vi "2011 Plotter Cole version.vi"() -> ()   [LabVIEW 2011]
uses:
  General-Controler/panel position.ctl
  shared programs/MySQL/Preset Query Enum.ctl
  plotter setup cluster.ctl
  <vilib>/Utility/tcp.llb/UDP Multicast Read-Only Open.vi
  <vilib>/Analysis/1siggen.llb/Ramp Pattern by Samples.vi
  <vilib>/Analysis/NI_AALBase.lvlib
panel:
  in  "STOP button":bool
  out "shot# 3":i32
  out "error out 3":errorcluster
  out "TCP Ports":refnum<k5>[](array[refnum])
  in  "Device name":string
  in  "shot #":i32
  in  "data string":string
  in  "data string 2":string
  in  "shot # 2":i32
  in  "Device name 2":string
  out "subscribe command":string
  out "size(s)":i32
  out "appended array":string[](array[string])
  out "y2":dbl[](array[numeric])
  out "y1":dbl[](array[numeric])
  out "error out 4":errorcluster
  out "x":dbl[](array[numeric])
  out "portrsvvv":string[](array[string])
  out "ipjjj":string[](array[string])
  out "IPs":string[](array[string])
  out "udp ports to listen to":string[](array[string])
  in  "TCP Open timeout ms":i32=1000
  out "TCP scan error out":errorcluster
  out "ScanData to receive":string[][](array[string])
  out "error out":errorcluster
  in  "Cluster":T1
  out "appargs":string[](array[string])
  out "plotter details":string[][](array[string])
  out "plotter#":string
  out "expt":string
  out "expt_plotter.id":string
  out "Mcast Data":string
  out "TDMS file path":path
  in  "Tab Control 2":T2(tab)
  out "parameters to get":string[][](array[string])
  out "devices to get data from":string[](array[string])
  out "Axis Name List":string[](array[string])
  out "All Devices Core Info":string[][](array[string])
  out "UDP Mcast Error":errorcluster
  in  "Tab Control":T3(tab)=enum."Binned Plot"
  out "xy graph":cluster{dbl[], dbl[]}[](graph)
  out "LHS sigma":dbl format="%_4p"
  out "LHS mean":dbl format="%_4p"
  out "RHS mean":dbl format="%_4p"
  out "RHS sigma":dbl format="%_4p"
  out "xy graph bin":cluster{dbl[], dbl[]}[](graph)=[{[5.5, 15.5, 25.5, 35.5, 45.5, 55.5, 0.0], [0.1, 0.1, 0.15, 0.15, 0.2, 0.2, 0.0]}, {[5.5, 5.5, nan, 15.5, 15.5, nan, 25.5, 25.5, nan, 35.5, 35.5, nan, 45.5, 45.5, nan, 55.5, 55.5, nan, 0.0, 0.0, nan], [0.1, 0.1, nan, 0.1, 0.1, nan, 0.15, 0.15, nan, 0.15, 0.15, nan, 0.2, 0.2, nan, 0.2, 0.2, nan, 0.0, 0.0, nan]}, {[5.5, 15.5, 25.5, 35.5, 45.5, 55.5, 0.0], [5.5, 15.5, 25.5, 35.5, 45.5, 55.5, 0.0]}, {[5.5, 5.5, nan, 15.5, 15.5, nan, 25.5, 25.5, nan, 35.5, 35.5, nan, 45.5, 45.5, nan, 55.5, 55.5, nan, 0.0, 0.0, nan], [3.0, 8.0, nan, 13.0, 18.0, nan, 23.0, 28.0, nan, 33.0, 38.0, nan, 43.0, 48.0, nan, 53.0, 58.0, nan, 0.0, 0.0, nan]}]
  in  "replot":bool
  out "Experiment":u16(ring) items=["10TW colliding pulse", "Bella", "FakeCam1only", "FakeCam1to5", "GOG", "Staging", "StagingTRA", "Test stand default", "TREX high power", "TREX low power"]
  out "Current State":string
  out "Mcast Path Data":string
  in  "FilePath":bool
  in  "file path":path
  in  "X Axis":u16(ring)=1 items=["FakeCam1 gain", "FakeCam2 gain", "FakeCam3 gain", "FakeCam4 gain", "FakeCam5 gain"]
  in  "Y Axis":u16(ring) items=["FakeCam1 gain", "FakeCam2 gain", "FakeCam3 gain", "FakeCam4 gain", "FakeCam5 gain"]
  in  "Y Axis 2":u16(ring) items=["FakeCam1 gain", "FakeCam2 gain", "FakeCam3 gain", "FakeCam4 gain", "FakeCam5 gain"]
  out "device data Spreadsheet format":string[][](array[string])
  in  "Left":i16=25
  in  "Top":i16=75
  in  "expt_Plotteridfor vi mode":string="17"
  in  "timeout ms":i32=1000
  out "x axis name":string
  out "ScanStart ExptName":string
  out "Y Axis Default name":string
  out "MC_IP":string
  out "Path used":path
  out "error out 2":errorcluster
  out "ScanStatus":string
  out "data out 1":string
  out "data out 3":string
  out "data out 2":string
  out "shotoverride":bool
  out "shot#":i32
  out "shot# 2":i32
  out "error out 5":errorcluster
  # "Plotter"
  # "17 Fake cam 1 to 5"
  # "15"
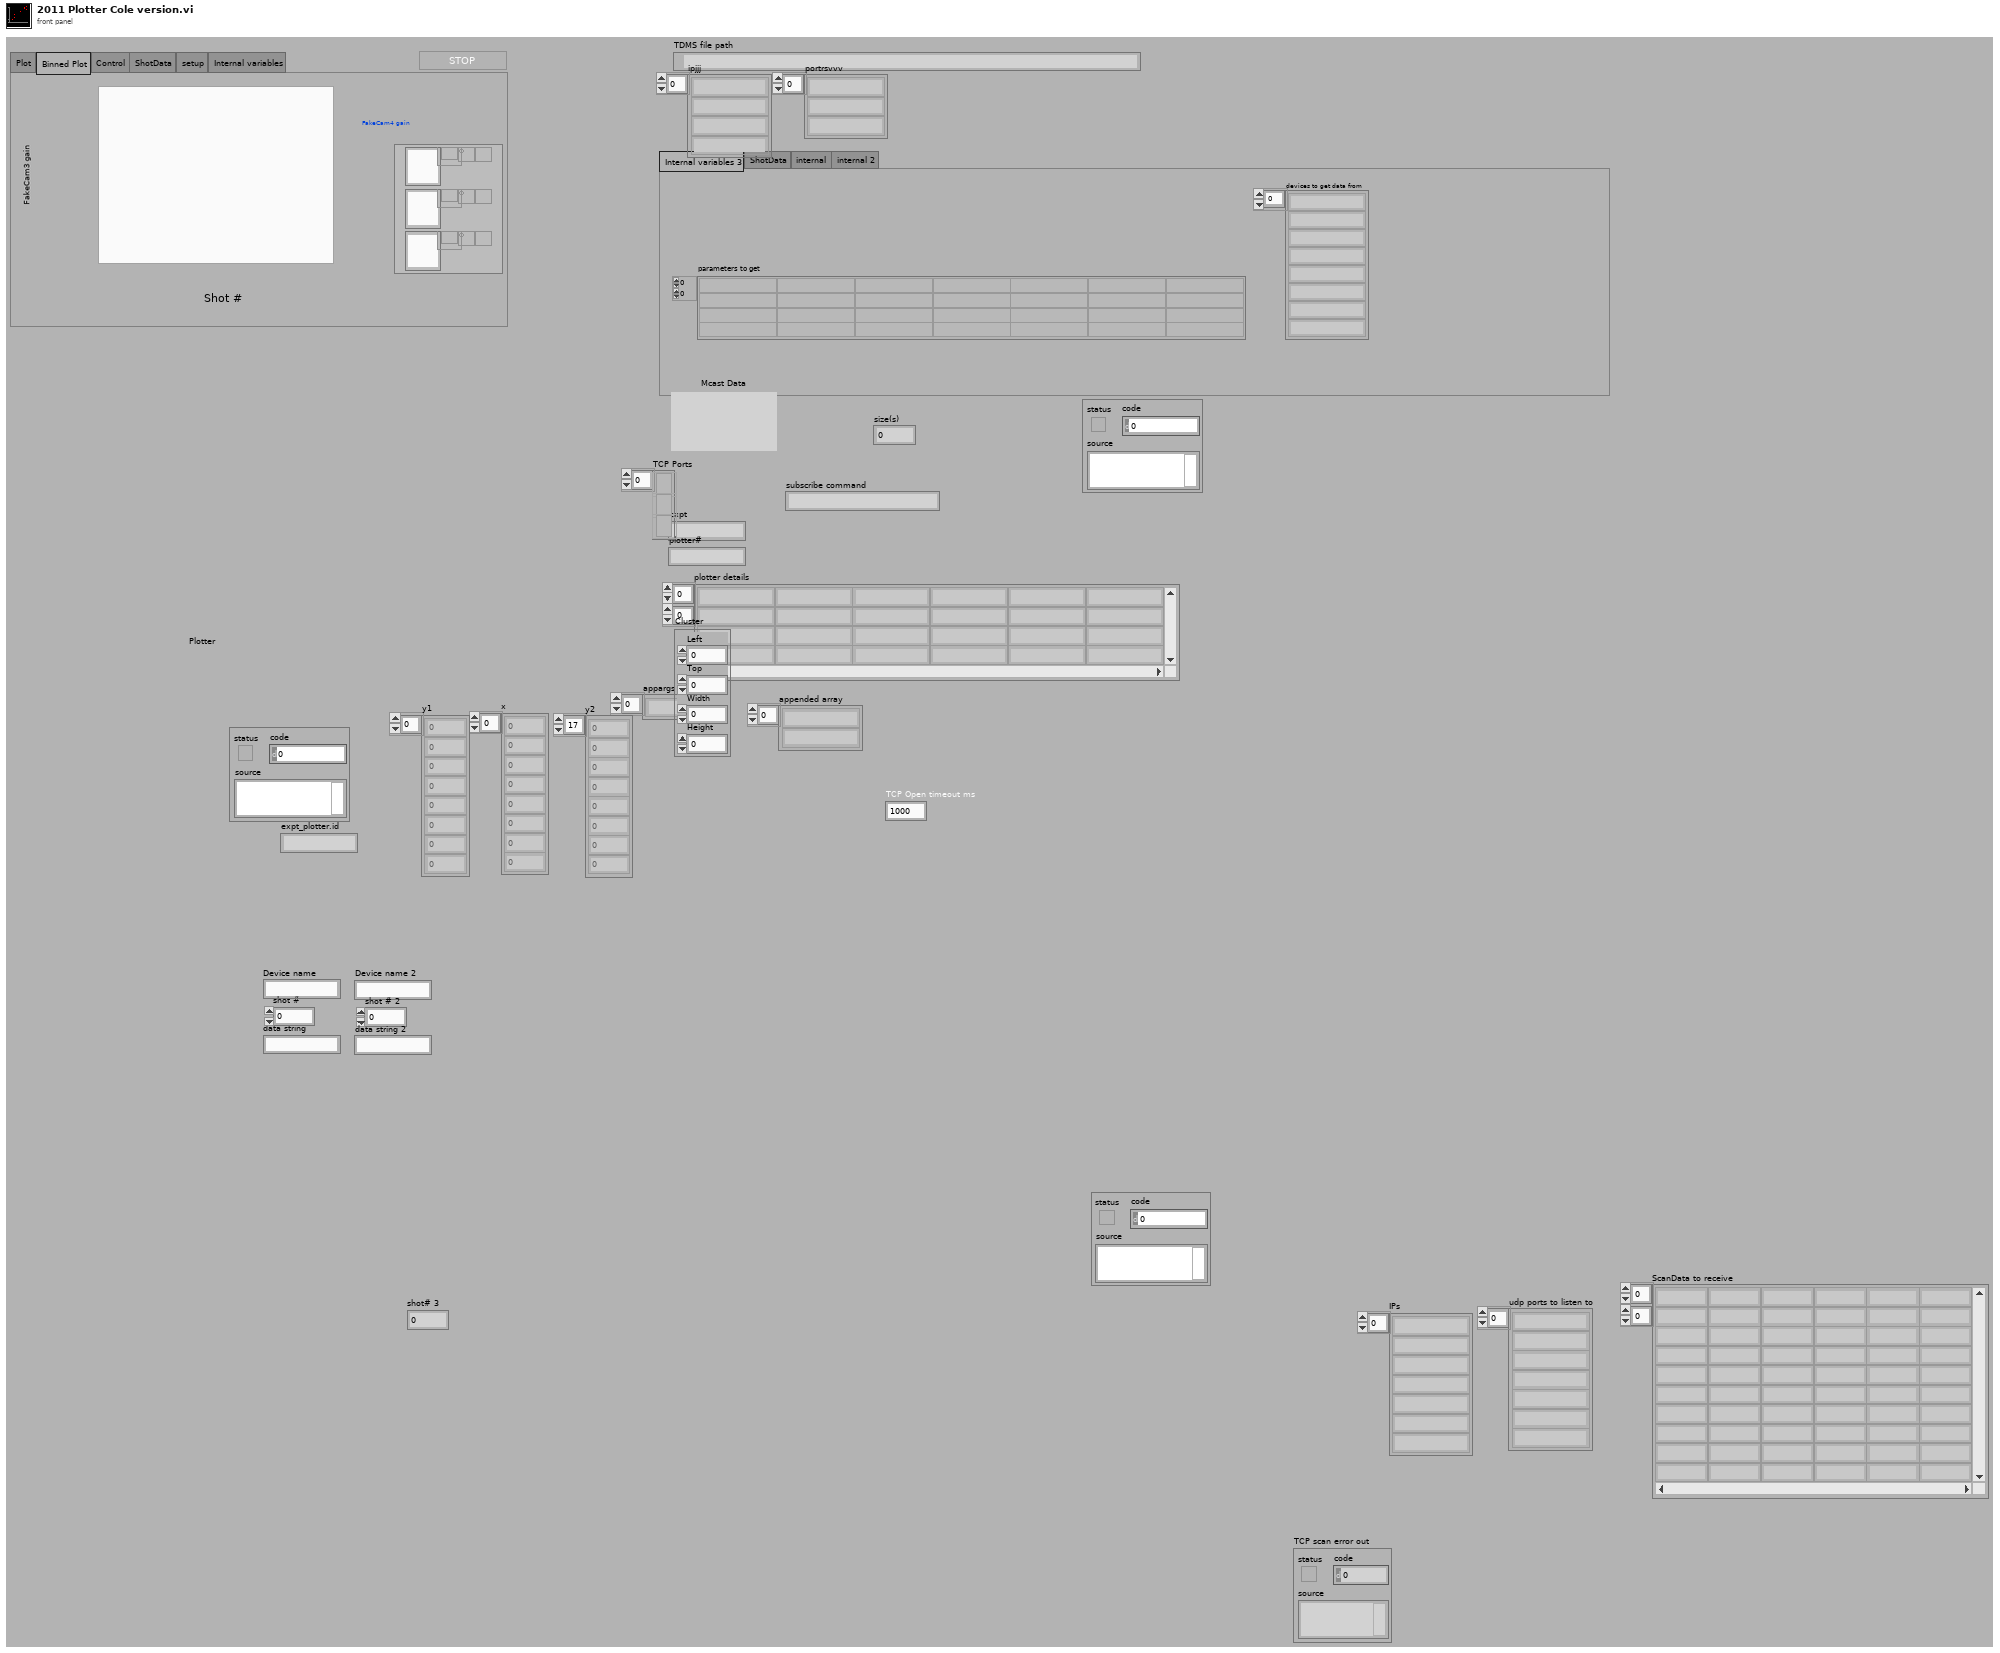
[diagram p1: front panel]
types:
  T1 = typedef "panel position.ctl" = cluster{"Left":i16, "Top":i16, "Width":u32, "Height":u32}
  T2 = enum32{"Internal variables 3", "ShotData", "internal", "internal 2"}
  T3 = enum32{"Plot", "Binned Plot", "Control", "ShotData", "setup", "Internal variables"}
  T4 = typedef "Plotter FGV cluster control.ctl" = cluster{"Multicast Address":string, "Plotter Busy":bool, "Plotter Exit":bool, "Mcast Port":u16}
  T5 = enum32{"invalid app kind", "Development System", "Run Time System", "Student Edition", "Embedded LabVIEW", "Evaluation", "Custom"}
  T6 = enum32{"Invalid", "Standard", "Closed", "Hidden", "Minimized", "Maximized"}
  T7 = typedef "Preset Query Enum.ctl" = enum16{"Get Locations", "Get all IPs and MACs", "Get classes", "Get expt variables to set at scanstart for particular device", "Get expt devices and variables with start values", "Get expt devices and variables (with data to get)", "Get expt devices with data to get", "Get Expt devices and GUIs", "Get all devices basic properties", "Get Virtual Devices Core Info", "Get Expt names", "Get experiment basic properties", "Get MC Ports", "Get device network comm port", "Get devicetype lvclass path", "Get basic device properties", "Get Init Order", "Get all setable variables of a device", "Get all variables of a devicetype", "Get all variables of a device", "Get plotter details", "Get expt for plotter", "Get plotter IDs from expt", "Get all devices", "Get all Virtual Devices", "Get variable and device info for Virtual Device", "GetItemLocatorIP", "Get IPs for GUIs", "Get DeviceType from Device"}
  T8 = typedef "plotter setup cluster.ctl" = cluster{"screenx":i16, "screeny":i16, "variable1":string, "variable2":string}
  T9 = cluster{"Ring Refnum x":refnum<vi>, "Ring Refnum y":refnum<vi>, "Ring Refnum y 2":refnum<vi>, "XY Graph Refnum":refnum<vi>}
  T10 = cluster{"Core":cluster{"Current VI Reference":refnum<vi>, "Close Panel on Exit?":bool}, "All Devices Core Info":string[][], "Expt Config Files":string[], "Experiment name":string, "ScanData to receive":string[][], "Device Names for scan data":string[], "expt config file array":string[][], "Data titles from config array":string[], "TDMS file path":path, "Plotter setup cluster":T8, "plotter#":string, "bin complete":bool}
  T11 = cluster{"TCP Ports":refnum<vi>, "y1":refnum<vi>, "shot#":refnum<vi>, "data out 1":refnum<vi>}
  T12 = cluster{"TCP Ports":refnum<vi>, "y2":refnum<vi>, "shot# 2":refnum<vi>, "data out 2":refnum<vi>}
  T13 = cluster{"TCP Ports":refnum<vi>, "x":refnum<vi>, "shot# 3":refnum<vi>, "data out 3":refnum<vi>}
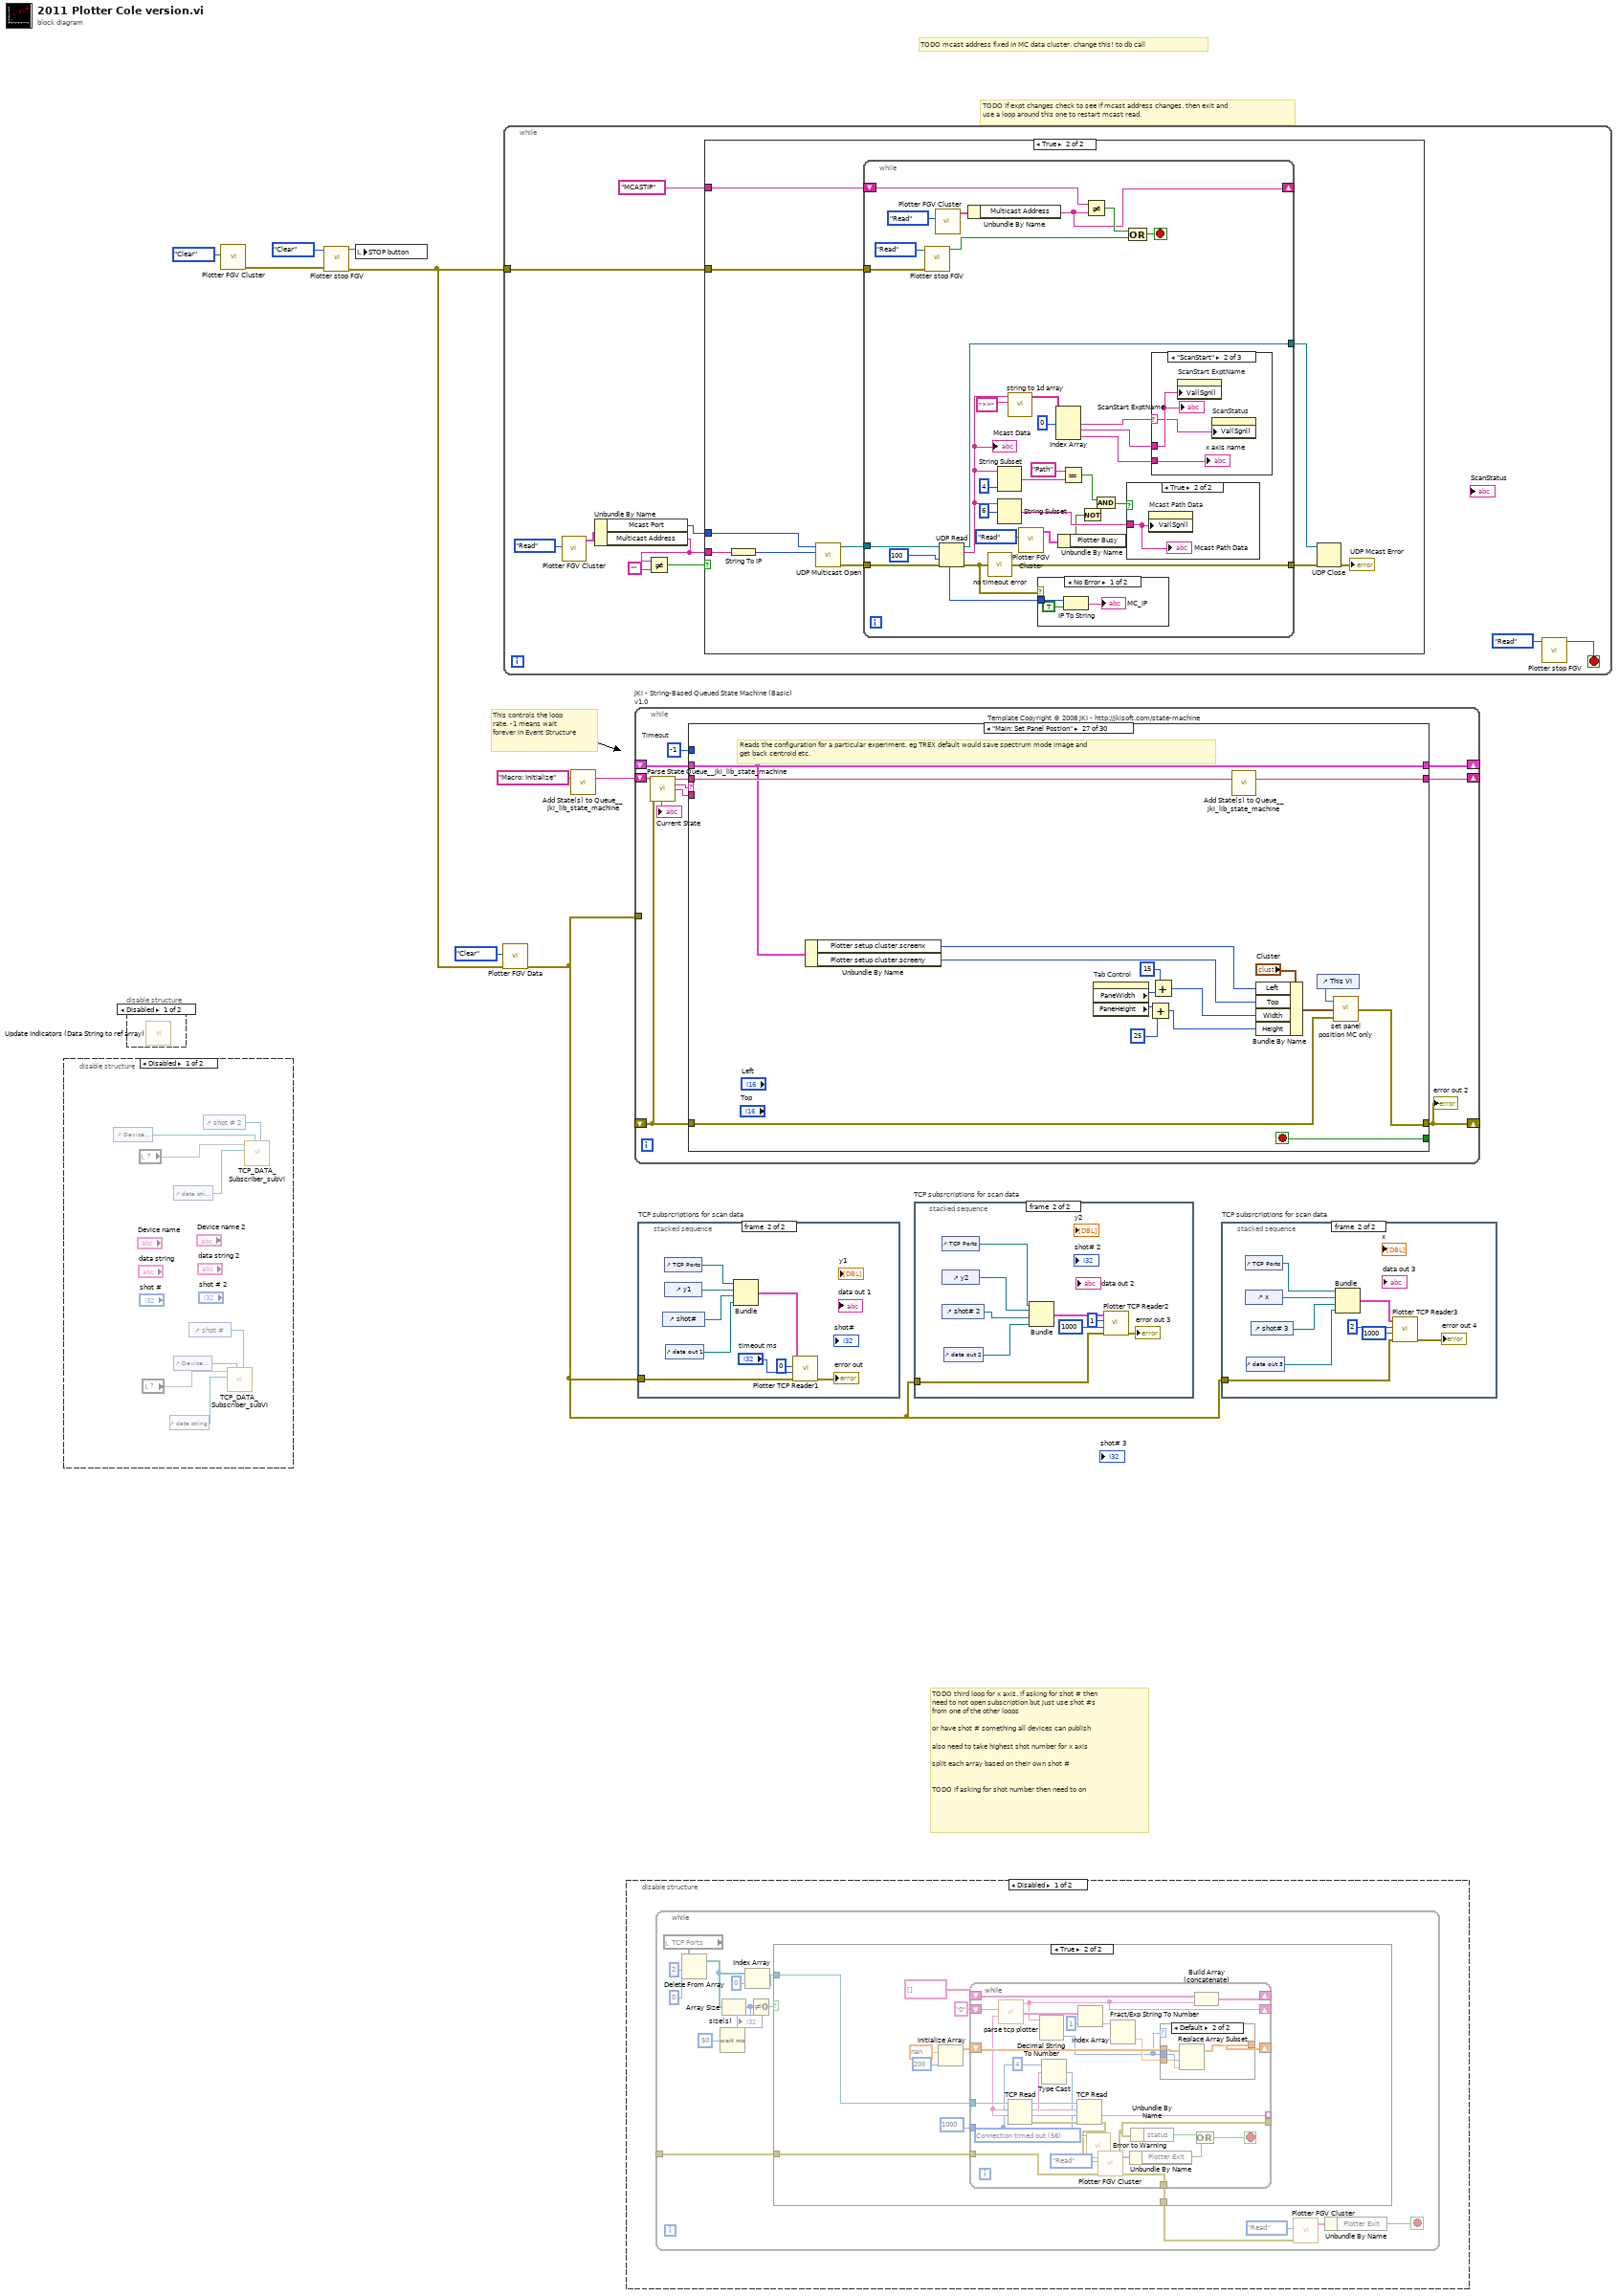
[diagram p0: block diagram]
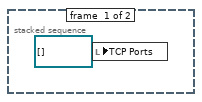
[diagram p5: hidden frame]
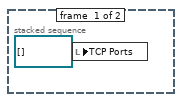
[diagram p6: hidden frame]
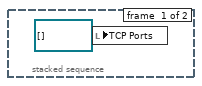
[diagram p8: hidden frame]
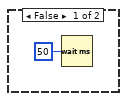
[diagram p10: hidden frame]
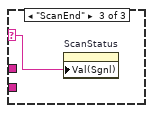
[diagram p14: hidden frame]
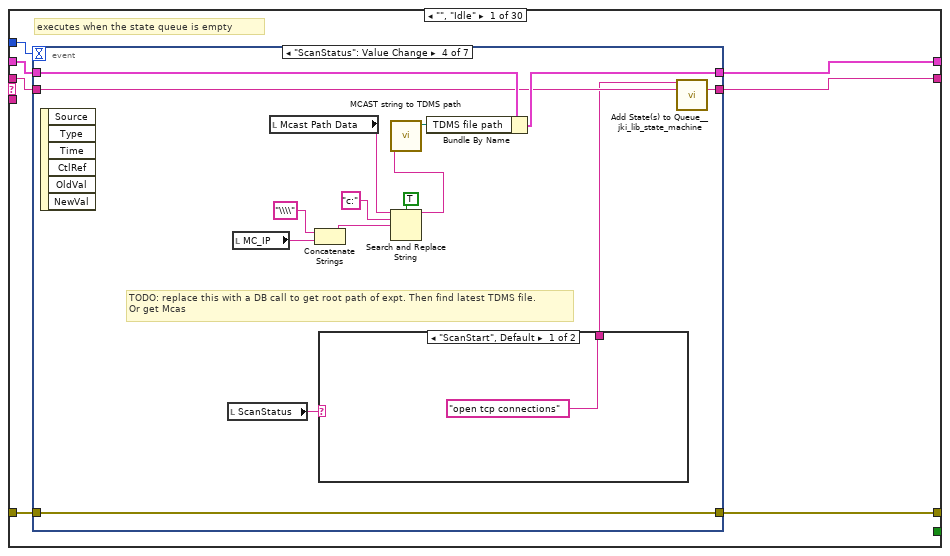
[diagram p15: hidden frame]
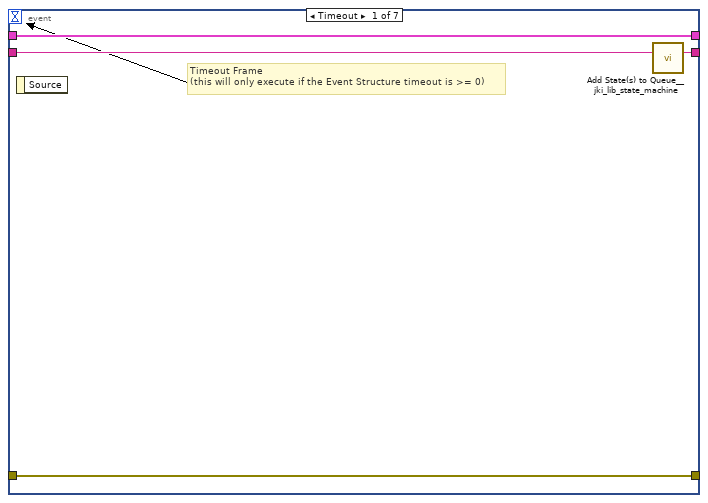
[diagram p16: hidden frame]
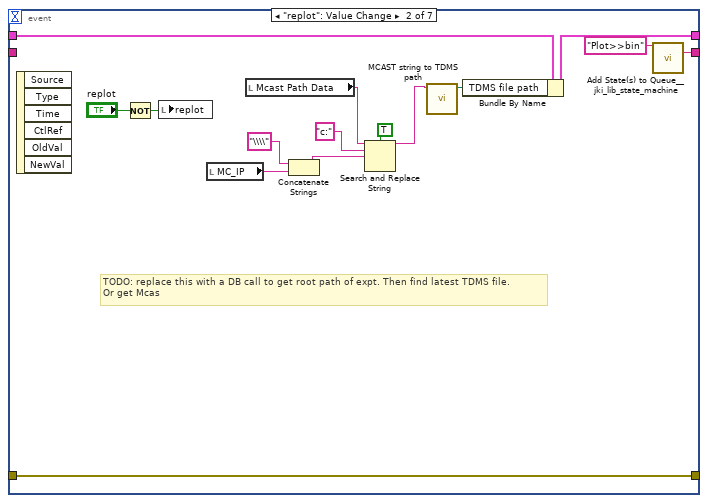
[diagram p17: hidden frame]
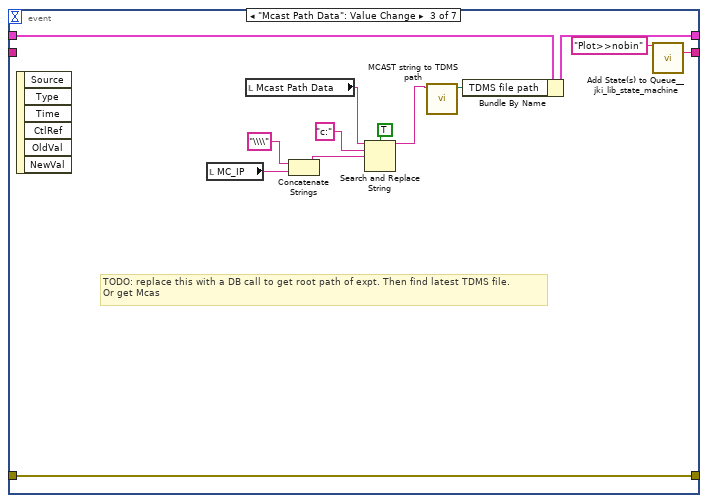
[diagram p18: hidden frame]
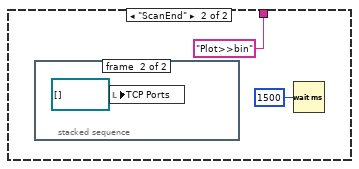
[diagram p19: hidden frame]
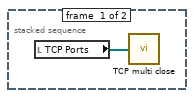
[diagram p20: hidden frame]
diagram:
  # "TODO third loop for x axis. if asking for shot # then \nneed to not open subscription but just use shot #s\nfrom one of the other loops\n\nor have shot # something all devices can publish\n\nalso need to take highest shot number for x axis\n\nsplit each array based on their own shot #\n\n\nTODO if asking for shot number then need to on"
  # "TODO mcast address fixed in MC data cluster. change this! to db call"
  # "TODO if expt changes check to see if mcast address changes. then exit and\nuse a loop around this one to restart mcast read."
  # "This controls the loop rate. -1 means wait forever in Event Structure"
  n1 = disable-structure shown="Disabled" {
    frame Disabled {
      n2 = control-ref of="Device name 2"() -> (w12:refnum<vi>)
      n3 = local read item#-1() -> (w10)
      n4 = local read item#-1() -> (w15)
      n5 = control-ref of="data string"() -> (w14:refnum<vi>)
      n6 = control-ref of="Device name"() -> (w17:refnum<vi>)
      n7 = control-ref of="data string 2"() -> (w11:refnum<vi>)
      n8 = control-ref of="shot #"() -> (w16:refnum<vi>)
      n9 = control-ref of="shot # 2"() -> (w13:refnum<vi>)
      n10 = call "TCP_DATA_Subscriber_subVi.vi"("shot number"=w16, "whatamI"=w17, 10:w14, "connection ID"=w15) -> ()  [unwired: 7 in, 1 out]
      n11 = call "TCP_DATA_Subscriber_subVi.vi"("shot number"=w13, "whatamI"=w12, 10:w11, "connection ID"=w10) -> ()  [unwired: 7 in, 1 out]
    }
    frame Enabled {
    }
  }
  n12 = disable-structure shown="Disabled" {
    frame Disabled {
      n13 = call "Update Indicators (Data String to ref array).vi"() -> ()  [unwired: 5 in, 1 out]
    }
    frame Enabled {
    }
  }
  n14 = call "Plotter FGV Cluster.vi"("Function"=enum16{"Read", "Write", "Clear"}."Clear") -> ("error out"=w5:errorcluster)  [unwired: 9 in, 1 out]
  n15 = call "Plotter stop FGV.vi"("error in"=w5, "Function"=enum16{"Read", "Write", "Clear"}."Clear") -> ("error out"=w2:errorcluster, "Stop out"=w4:bool)  [unwired: 8 in]
  n16 = local write "STOP button"(w4) -> ()
  n17 = call "Plotter FGV Data.vi"("error in"=w2, "Function"=enum16{"Read", "Write", "Clear"}."Clear") -> ("error out"=w1:errorcluster)  [unwired: 8 in, 1 out]
  n18 = while {
    tunnel: w2 -> [w21]
    stop <- w25 stop-if-true
    n19 = call "Plotter FGV Cluster.vi"("Function"=enum16{"Read", "Write", "Clear"}."Read") -> ("Cluster out"=w22:T4)  [unwired: 9 in, 1 out]
    n20 = Unbundle By Name(w22) -> ("Mcast Port"=w18:u16, "Multicast Address"=w20:string)
    n21 = Not Equal?(x=w20, y="") -> (x != y?=w24:bool)
    n22 = case shown="True" w24 {
      tunnel: "MCASTIP" ("Multicast Address") -> [_ w32]
      tunnel: w20 -> [_ w31]
      tunnel: w21 -> [_ w30]
      tunnel: w18 -> [_ w29]
      frame False {
        n23 = Wait (ms)(milliseconds to wait=u32 50) -> ()  [unwired: 1 out]
      }
      frame True {
        n24 = String To IP(1:w31) -> (0:w38:u32)
        n25 = call-poly <vilib>:"UDP Multicast Open.vi"("multicast addr"=w38, "port"=w29) -> ("error out"=w33:errorcluster, "connection ID"=w37:refnum<k16>)  [unwired: 7 in, 1 out]
        n26 = while {
          tunnel: w37 -> [w71]
          tunnel: [w70] -> w36
          tunnel: [w69] -> w35
          tunnel: w33 -> [w65]
          tunnel: w30 -> [w63]
          shift-right: [w39] -> _
          shift-left: w32 -> [w51]
          stop <- w52 stop-if-true
          n27 = call "Plotter stop FGV.vi"("error in"=w63, "Function"=enum16{"Read", "Write", "Clear"}."Read") -> ("Stop out"=w53:bool)  [unwired: 8 in, 1 out]
          n28 = call "Plotter FGV Cluster.vi"("Function"=enum16{"Read", "Write", "Clear"}."Read") -> ("Cluster out"=w50:T4)  [unwired: 9 in, 1 out]
          n29 = UDP Read(connection ID=w71, timeout ms (25000)=100, 8:w65) -> (data out=w54:string, error out=w41:errorcluster, 3:w70:refnum<k16>, 6:w42:u32)  [unwired: 2 out]
          "Mcast Data" <- w54
          n30 = Unbundle By Name(w50) -> ("Multicast Address"=w39:string)
          n31 = call "no timeout error.vi"("error in (no error)"=w41) -> ("error out"=w69:errorcluster)
          n32 = String Subset(string=w54, length (rest)=4 ("length (rest)")) -> (substring=w60:string)  [unwired: 1 in]
          n33 = String Subset(string=w54, offset (0)=6) -> (substring=w58:string)  [unwired: 1 in]
          n34 = call "string to 1d array.vi"("delimiter (Tab)"=">>", "string"=w54) -> ("Array of Strings"=w67:string[])  [unwired: 9 in]
          n35 = call "Plotter FGV Cluster.vi"("Function"=enum16{"Read", "Write", "Clear"}."Read") -> ("Cluster out"=w45:T4)  [unwired: 9 in, 1 out]
          n36 = case shown="No Error" w41 {
            tunnel: w42 -> [w75 _]
            frame No Error {
              n37 = IP To String(1:TRUE ("dot notation? (F)"), 2:w75) -> (0:→"MC_IP":string)
            }
            frame Error {
            }
          }
          n38 = Index Array(array=w67, index #1=0 ("index")) -> (element #1=w48:string, element #2=w55:string, element #3=w56:string)  [unwired: 2 in]
          n39 = Unbundle By Name(w45) -> ("Plotter Busy"=w44:bool)
          n40 = Equal?(x="Path" ("y"), y=w60) -> (x = y?=w57:bool)
          n41 = Not(x=w44) -> (.not. x?=w43:bool)
          n42 = Not Equal?(x=w51, y=w39) -> (x != y?=w40:bool)
          n43 = And(x=w57, y=w43) -> (x .and. y?=w47:bool)
          n44 = case shown="True" w47 {
            tunnel: w58 -> [_ w76]
            frame False {
            }
            frame True {
              n45 = property on="Mcast Path Data" class="Str"("Val(Sgnl)"=w76) -> ()  [unwired: 2 in, 2 out]
              "Mcast Path Data" <- w76
            }
          }
          n46 = Compound Arithmetic op=OR(w40, w53) -> (w52:bool)
          n47 = case shown="\"ScanStart\"" w48 {
            selector: w48 -> [_ w77 w80]
            tunnel: w56 -> [_ w79 _]
            tunnel: w55 -> [_ w78 _]
            frame Default {
            }
            frame "ScanStart" {
              n48 = property on="ScanStart ExptName" class="Str"("Val(Sgnl)"=w78) -> ()  [unwired: 2 in, 2 out]
              n49 = property on="ScanStatus" class="Str"("Val(Sgnl)"=w77) -> ()  [unwired: 2 in, 2 out]
              "x axis name" <- w79
              "ScanStart ExptName" <- w78
            }
            frame "ScanEnd" {
              n50 = property on="ScanStatus" class="Str"("Val(Sgnl)"=w80) -> ()  [unwired: 2 in, 2 out]
            }
          }
        }
        n51 = UDP Close(connection ID=w36, 8:w35) -> (error out=→"UDP Mcast Error":errorcluster)  [unwired: 1 out]
      }
    }
    n52 = call "Plotter stop FGV.vi"("Function"=enum16{"Read", "Write", "Clear"}."Read") -> ("Stop out"=w25:bool)  [unwired: 9 in, 1 out]
  }
  n53 = call <vilib>:"Add State(s) to Queue__jki_lib_state_machine.vi"("State(s) in (\"\")"="Macro: Initialize") -> ("States Out"=w9:string)  [unwired: 14 in]
  n54 = disable-structure shown="Disabled" {
    frame Disabled {
      n55 = while {
        tunnel: _ -> [w87]
        stop <- w88 stop-if-true
        n56 = local read "TCP Ports"() -> (w91:refnum<k5>[])
        n57 = Delete From Array(array=w91, length=2, index=0) -> (array with subset deleted=w83:refnum<k5>[])  [unwired: 1 out]
        n58 = Wait (ms)(milliseconds to wait=u32 50) -> ()  [unwired: 1 out]
        n59 = Array Size(array=w83) -> (size(s)=w94:i32)
        "size(s)" <- w94
        n60 = Index Array(array=w83, index=0) -> (element=w86:refnum<k5>)
        n61 = Not Equal To 0?(x=w94) -> (x != 0?=w93:bool)
        n62 = case shown="True" w93 {
          tunnel: w86 -> [_ w102]
          tunnel: w87 -> [_ w101]
          tunnel: [_ w100] -> w81
          frame False {
          }
          frame True {
            n63 = Initialize Array(nan ("element"), 200 ("dimension size")) -> (w95:dbl[])
            n64 = while {
              tunnel: [w113] -> _
              tunnel: w102 -> [w131]
              tunnel: 1000 ("timeout ms 3") -> [w129]
              tunnel: [w104] -> _ mode=indexing
              shift-right: [w112] -> _
              shift-left: "0" ("shot #") -> [w123]
              tunnel: w101 -> [w119]
              tunnel: [w118] -> w100
              shift-right: [w110] -> _
              shift-left: string[] [] -> [w111]
              shift-right: [w106] -> _
              shift-left: w95 -> [w108]
              stop <- w125 stop-if-true
              w115 = 56 items=["No Error", "Argument Error", "Memory Full", "Out of Zone", "End of File", "File Already Open", "Generic File IO Error", "File Not Found", "File Permission Error", "Disk Full", "Duplicate Path", "Too Many Files Open", "Not Enabled", "Resource File Not Found", "Cannot Add Resource", "Resource Not Found", "Image Not Found", "Image Memory Error", "Pen Does Not Exist", "Config Bad Type", "Config Token Not Found", "Config Parse Error", "Config Memory Error", "Bad External Code Format", "Bad External Code Offset", "External Code Not Present", "Null Window", "Destroy Window Mixup", "Null Menu", "Print Aborted", "Bad Print Record", "Print Driver Error", "Windows Error During Print", "Memory Error During Print", "Print Dialog Error", "Generic Print Error", "Invalid Device Refnum", "Device Not Found", "Device Parameter Error", "Device Unit Error", "Can't Open Device", "Device Call Aborted", "Generic Error", "Cancelled By User", "Object ID Too Low", "Object ID Too High", "Object Not In Heap", "Unknown Heap", "Bad DefProc ID", "DefProc Not In Table", "Message Out Of Range", "Null Method", "Unknown Message", "Manager Call Not Supported", "Bad address", "Connection In progress", "Connection timed out", "Connection is already in progress", "Network attribute not supported", "Network error", "Address in use", "System out of memory", "Connection aborted", "Connection refused", "Connection is not connected", "Connection is already connected", "Connection closed", "Initialize error (interapplication manager)", "Bad occurrence", "Wait on unbound occurrence handler", "Occurrence queue overflow", "Bad path", "Semaphore not signaled", "Unrecognized type (interapplication manager)"] ("1st Error to Convert")
              w128 = 4 ("bytes to read")
              n65 = TCP Read(connection ID=w131, bytes to read=w128, 9:w129) -> (connection ID out=w132:refnum<k5>, data out=w127:string, error out=w130:errorcluster)  [unwired: 2 in]
              n66 = Type Cast(type=w128, x=w127) -> (*(type *) &x=w126:i32)
              n67 = TCP Read(connection ID=w132, bytes to read=w126, error in (no error)=w130, 9:w129) -> (data out=w104:string, error out=w114:errorcluster)  [unwired: 1 in, 1 out]
              n68 = call "parse tcp plotter.vi"("data in"=w104, "shot #"=w123) -> ("variable values"=w117:string[], "shot # out"=w112:string)  [unwired: 8 in]
              n69 = Decimal String To Number(string=w112) -> (number=w105:i32)  [unwired: 2 in, 1 out]
              n70 = Index Array(array=w117, index=1) -> (element=w116:string)
              n71 = call <vilib>:"Error to Warning.vi"("1st Error to Convert"=w115, "error in"=w114) -> ("warning out"=w113:errorcluster)  [unwired: 13 in]
              n72 = call "Plotter FGV Cluster.vi"("error in"=w119, "Function"=enum16{"Read", "Write", "Clear"}."Read") -> ("error out"=w118:errorcluster, "Cluster out"=w121:T4)  [unwired: 8 in]
              n73 = Fract/Exp String To Number(string=w116) -> (number=w107:dbl)  [unwired: 3 in, 1 out]
              n74 = Unbundle By Name(w121) -> ("Plotter Exit"=w120:bool)
              n75 = Unbundle By Name(w113) -> ("status"=w124:bool)
              n76 = case shown="Default" w105 {
                tunnel: w108 -> [w133 w137]
                tunnel: w105 -> [_ w136]
                tunnel: w107 -> [_ w135]
                tunnel: [w133 w134] -> w106
                frame 0 {
                }
                frame Default {
                  n77 = Replace Array Subset(array=w137, new element=w135, index=w136) -> (w134:dbl[])
                }
              }
              n78 = Or(x=w124, y=w120) -> (x .or. y?=w125:bool)
              n79 = Build Array (concatenate)(w111, w112) -> (w110:string[])
            }
          }
        }
        n80 = call "Plotter FGV Cluster.vi"("error in"=w81, "Function"=enum16{"Read", "Write", "Clear"}."Read") -> ("Cluster out"=w90:T4)  [unwired: 8 in, 1 out]
        n81 = Unbundle By Name(w90) -> ("Plotter Exit"=w88:bool)
      }
    }
    frame Enabled {
    }
  }
  n82 = while "JKI - String-Based Queued State Machine (Basic) v1.0" {
    shift-right: [w142] -> _
    shift-left: _ -> [w141]
    shift-right: [w138] -> _
    shift-left: _ -> [w139]
    shift-right: [w144] -> _
    shift-left: w9 -> [w145]
    tunnel: w1 -> [_]
    stop <- w143 stop-if-true
    w140 = -1  # Timeout
    # "Template Copyright © 2008 JKI - http://jkisoft.com/state-machine"
    n83 = call <vilib>:"Parse State Queue__jki_lib_state_machine.vi"("State Queue"=w145, "Error In (no error)"=w139) -> ("Remaining States"=w147:string, "Current State"=w148:string, "Arguments"=w146:string)  [unwired: 11 in]
    "Current State" <- w148
    n84 = case shown="\"Main: Set Panel Postion\"" w148 {
      selector: w148 -> [_ _ _ w247 _ _ _ _ _ _ _ _ _ _ _ _ _ _ _ _ _ _ _ _ _ _ _ _ _ _]
      tunnel: w147 -> [w155 w242 w246 w251 w269 w276 w281 w285 w289 w295 w299 w303 w309 w320 w346 w351 w361 w365 w371 w380 w400 w428 w457 w470 w486 w501 w574 w582 w607 w694]
      tunnel: w146 -> [_ _ _ _ _ _ _ _ _ _ _ _ w304 w314 _ _ _ _ _ _ _ _ _ _ _ _ _ _ w584 _]
      tunnel: w141 -> [w153 w239 w243 w249 w260 w273 w279 w282 _ w290 w296 w301 w307 w316 w343 w347 w359 w362 w368 w377 w398 w414 w455 w463 w483 w499 w568 w579 w605 w691]
      tunnel: [w152 w240 w244 w253 w266 errorcluster {"status"=FALSE, "code"=0, "source"=""} ("error out") w278 w283 w287 w291 w297 w300 w305 w317 w344 w349 w352 w363 w369 w372 w386 w410 w446 w468 w484 w497 w559 w575 w585 w692] -> w138
      tunnel: w139 -> [w151 w240 w244 w252 w266 w270 w278 w283 w287 w292 w297 w300 w306 w318 w344 w349 w352 w363 w369 w373 w387 w411 w436 w468 w484 w498 w560 w576 w586 w692]
      tunnel: [w154 w241 w245 w250 w268 w275 w280 w284 w288 w294 w298 w302 w308 w319 w345 w350 w360 w364 w370 w379 w399 w427 w456 w469 w485 w500 w573 w581 w606 w693] -> w144
      tunnel: [_ _ _ _ _ _ TRUE _ _ _ _ _ _ _ _ _ _ _ _ _ _ _ _ _ _ _ _ _ _ _] -> w143
      tunnel: [w150 w239 w243 w249 w267 w273 w279 w282 w286 w290 w296 w301 w307 w316 w343 w347 w359 w362 w368 w376 w397 w413 w454 w462 w483 w499 w568 w580 w605 w691] -> w142
      tunnel: w140 -> [w149 _ _ _ _ _ _ _ _ _ _ _ _ _ _ _ _ _ _ _ _ _ _ _ _ _ _ _ _ _]
      frame "", "Idle" {
        # "executes when the state queue is empty"
        n85 = event shown="[3] \"ScanStatus\": Value Change" {
          selector: _ -> [_ _ _ _ _ _ _]
          dyn-events: _ -> [_ _ _ _ _ _ _]
          timeout: w149 -> [_ _ _ _ _ _ _]
          tunnel: w155 -> [w159 _ _ w197 w218 w232 w238]
          tunnel: [w158 w174 w187 w202 w217 w231 w237] -> w154
          tunnel: w153 -> [w156 w171 w184 w200 w209 w229 w235]
          tunnel: [w157 w173 w186 w201 w216 w230 w236] -> w152
          tunnel: w151 -> [w157 w173 w186 w201 w216 w230 w236]
          tunnel: [w156 w170 w183 w199 w208 w229 w235] -> w150
          event Timeout {
            # "Timeout Frame\n(this will only execute if the Event Structure timeout is >= 0)"
            n86 = event-data() -> ()  [unwired: 1 in, 1 out]
            n87 = call <vilib>:"Add State(s) to Queue__jki_lib_state_machine.vi"("State(s) in (\"\")"=w159) -> ("States Out"=w158:string)  [unwired: 14 in]
          }
          event "replot": Value Change {
            # "TODO: replace this with a DB call to get root path of expt. Then find latest TDMS file.\nOr get Mcas"
            n88 = event-data() -> ()  [unwired: 1 in, 6 out]
            n89 = Not(x="replot") -> (.not. x?=w168:bool)
            n90 = local write "replot"(w168) -> ()
            n91 = local read "MC_IP"() -> (w164:string)
            n92 = local read "Mcast Path Data"() -> (w166:string)
            n93 = Concatenate Strings("\\\\" ("string"), w164) -> (w161:string)
            n94 = Search and Replace String(case sensitive?=TRUE ("ignore case? (F)"), input string=w166, search string="c:" ("string"), replace string=w161) -> (result string=w160:string)  [unwired: 4 in, 3 out]
            n95 = call "MCAST string to TDMS path.vi"("MCAST path"=w160) -> ("TDMS path"=w167:path)  [unwired: 10 in]
            n96 = Bundle By Name(cluster=w171, "TDMS file path"=w167) -> (w170:T10)
            n97 = call <vilib>:"Add State(s) to Queue__jki_lib_state_machine.vi"("State(s) in Front (\"\")"="Plot>>bin" ("State(s) in Front (\"\")")) -> ("States Out"=w174:string)  [unwired: 14 in]
          }
          event "Mcast Path Data": Value Change {
            # "TODO: replace this with a DB call to get root path of expt. Then find latest TDMS file.\nOr get Mcas"
            n98 = event-data() -> ()  [unwired: 1 in, 6 out]
            n99 = local read "MC_IP"() -> (w179:string)
            n100 = local read "Mcast Path Data"() -> (w181:string)
            n101 = Concatenate Strings("\\\\" ("string"), w179) -> (w176:string)
            n102 = Search and Replace String(case sensitive?=TRUE ("ignore case? (F)"), input string=w181, search string="c:" ("string"), replace string=w176) -> (result string=w175:string)  [unwired: 4 in, 3 out]
            n103 = call "MCAST string to TDMS path.vi"("MCAST path"=w175) -> ("TDMS path"=w182:path)  [unwired: 10 in]
            n104 = Bundle By Name(cluster=w184, "TDMS file path"=w182) -> (w183:T10)
            n105 = call <vilib>:"Add State(s) to Queue__jki_lib_state_machine.vi"("State(s) in Front (\"\")"="Plot>>nobin" ("State(s) in Front (\"\")")) -> ("States Out"=w187:string)  [unwired: 14 in]
          }
          event "ScanStatus": Value Change {
            # "TODO: replace this with a DB call to get root path of expt. Then find latest TDMS file.\nOr get Mcas"
            n106 = event-data() -> ()  [unwired: 1 in, 6 out]
            n107 = local read "ScanStatus"() -> (w189:string)
            n108 = local read "MC_IP"() -> (w195:string)
            n109 = local read "Mcast Path Data"() -> (w191:string)
            n110 = Concatenate Strings("\\\\" ("string"), w195) -> (w192:string)
            n111 = case shown="\"ScanStart\", Default" w189 {
              tunnel: ["open tcp connections" ("State(s) in Front (\"\")") "Plot>>bin" ("State(s) in Front (\"\")")] -> w188
              frame "ScanStart", Default {
              }
              frame "ScanEnd" {
                n112 = stacked-sequence {
                  frame #0 {
                    n113 = local read "TCP Ports"() -> (w206:refnum<k5>[])
                    n114 = call "TCP multi close.vi"("TCP Ports"=w206) -> ()
                  }
                  frame #1 {
                    n115 = local write "TCP Ports"(refnum<k5>[] [] ("TCP Ports")) -> ()
                  }
                }
                n116 = Wait (ms)(milliseconds to wait=u32 1500) -> ()  [unwired: 1 out]
              }
            }
            n117 = Search and Replace String(case sensitive?=TRUE ("ignore case? (F)"), input string=w191, search string="c:" ("string"), replace string=w192) -> (result string=w190:string)  [unwired: 4 in, 3 out]
            n118 = call "MCAST string to TDMS path.vi"("MCAST path"=w190) -> ("TDMS path"=w198:path)  [unwired: 10 in]
            n119 = Bundle By Name(cluster=w200, "TDMS file path"=w198) -> (w199:T10)
            n120 = call <vilib>:"Add State(s) to Queue__jki_lib_state_machine.vi"("State(s) in Front (\"\")"=w188, "State(s) in (\"\")"=w197) -> ("States Out"=w202:string)  [unwired: 13 in]
          }
          event "ScanStart ExptName": Value Change {
            w211 = dbl[] [] ("y1")
            n121 = event-data() -> ()  [unwired: 1 in, 6 out]
            n122 = Bundle By Name(cluster=w209, "bin complete"=FALSE) -> (w208:T10)
            n123 = local read "ScanStart ExptName"() -> (w213:string)
            n124 = property on="Experiment" class="Ring (strict)"() -> ("Strings []"=w214:string[])  [unwired: 2 in, 2 out]
            n125 = Search 1D Array(1D array=w214, element=w213) -> (index of element=w212:i32)  [unwired: 1 in]
            n126 = local write "y2"(w211) -> ()
            n127 = local write "y1"(w211) -> ()
            n128 = local write "x"(w211) -> ()
            n129 = local write "Experiment"(w212) -> ()
            n130 = call <vilib>:"Add State(s) to Queue__jki_lib_state_machine.vi"("State(s) in Front (\"\")"="Main: Macro", "State(s) in (\"\")"=w218) -> ("States Out"=w217:string)  [unwired: 13 in]
          }
          event "STOP button": Value Change {
            # "Exit Button Value Change (pressed) Event\n(this executes Macro: Exit to terminate the VI)"
            n131 = event-data() -> ()  [unwired: 1 in, 1 out]
            n132 = call "Plotter stop FGV.vi"("Stop in"="STOP button", "Function"=enum16{"Read", "Write", "Clear"}."Write") -> ("Stop out"=w226:bool)  [unwired: 8 in, 1 out]
            n133 = Not(x=w226) -> (.not. x?=w225:bool)
            n134 = call "Plotter FGV Cluster.vi"("Function"=enum16{"Read", "Write", "Clear"}."Read") -> ("Cluster out"=w221:T4)  [unwired: 9 in, 1 out]
            n135 = Bundle By Name(cluster=w221, "Plotter Exit"=TRUE) -> (w219:T4)
            n136 = local write "STOP button"(w225) -> ()
            n137 = call "Plotter FGV Cluster.vi"("Function"=enum16{"Read", "Write", "Clear"}."Write", "Cluster in"=w219) -> ()  [unwired: 8 in, 2 out]
            n138 = call <vilib>:"Add State(s) to Queue__jki_lib_state_machine.vi"("State(s) in Front (\"\")"="Macro: Exit", "State(s) in (\"\")"=w232) -> ("States Out"=w231:string)  [unwired: 13 in]
          }
          event Panel Close? {
            # "Discard the event because we'll close the front panel ourselves in Macro: Exit"
            # "Close Panel button (pressed) Event\n(this executes Macro: Exit to terminate the VI)"
            n139 = event-data() -> ()  [unwired: 1 in, 1 out]
            n140 = event-data("Discard?"=TRUE) -> ()  [unwired: 1 in, 1 out]
            n141 = call <vilib>:"Add State(s) to Queue__jki_lib_state_machine.vi"("State(s) in Front (\"\")"="Macro: Exit", "State(s) in (\"\")"=w238) -> ("States Out"=w237:string)  [unwired: 13 in]
          }
        }
      }
      frame "Readme" {
        # "For instructions on how to use the JKI State Machine, examples and video tutorials, visit:\nhttp://jkisoft.com/state-machine/\n\nJKI State Machine™\nhttp://jkisoft.com/state-machine/\nCopyright (C) 2005-2008, JKI <info@jkisoft.com>\nALL RIGHTS RESERVED"
        # "copy this to create labels for wires"
        # "System_Label"
        # "State Syntax:\nStateCategory: State >> Argument\nLine Terminator: Line feed\nExample:\nUI: Help >> About\n\nWhere \"UI\" is the state category\nWhere \"Help\" is the state\nWhere \"About\" is the argument\nOther Examples:\nApp Data: Initialize\nUI: Initialize\nHelp >> About\n\nCommenting:\nTo add a comment use \"//\" or \"#\" and all text to the right will be ignored\nCommenting Example:\nUI: Initialize // This initializes the UI\n# This whole line is a comment\n// Another comment line"
        # "Readme"
        n142 = call <vilib>:"Add State(s) to Queue__jki_lib_state_machine.vi"("State(s) in (\"\")"=w242) -> ("States Out"=w241:string)  [unwired: 14 in]
      }
      frame "---------- Core ----------" {
        # "Do not put any code in this frame.\n(it is a separator no-op)"
        n143 = call <vilib>:"Add State(s) to Queue__jki_lib_state_machine.vi"("State(s) in (\"\")"=w246) -> ("States Out"=w245:string)  [unwired: 14 in]
      }
      frame Default {
        w256 = 42 items=["No error", "Argument error", "Memory is full", "Out of zone", "End of file", "File already open", "Generic file I/O error", "File not found", "File permission error", "Disk is full", "Duplicate path", "Too many files open", "System feature not enabled", "Resource file not found", "Cannot add resource", "Resource not found", "Image not found", "Image memory error", "Pen does not exist", "Config type invalid", "Config token not found", "Config parse error", "Config memory error", "Bad external code format", "Bad external code offset", "External code not present", "Null window", "Destroy window error", "Null menu", "Print aborted", "Bad print record", "Print driver error", "Windows error during printing", "Memory error during printing", "Print dialog error", "Generic print error", "Invalid device refnum", "Device not found", "Device parameter error", "Device unit error", "Cannot open device", "Device call aborted", "Generic error", "Cancelled by user", "Object ID too low", "Object ID too high", "Object not in heap", "Unknown heap", "Unknown object (invalid DefProc)", "Unknown object (DefProc not in table)", "Message out of range", "Invalid (null) method", "Unknown message", "Manager call not supported", "Bad address", "Network operation in progress", "Network operation timed out", "Connection is busy", "Network attribute not supported", "Network error", "Address in use", "System out of memory", "Connection aborted", "Connection refused", "Not connected", "Already connected", "Connection closed", "Initialization error (interapplication manager)", "Bad occurrence", "Wait on unbound occurrence handler", "Occurrence queue overflow", "Datalog type conflict", "Unused", "Unrecognized type (interapplication manager)", "Memory corrupt", "Failed to make temporary DLL", "Old CIN version", "Drag socket not found", "Failed to load drop-object", "Failed to register OLE object", "Failed to release OLE object", "Format specifier type mismatch", "Unknown format specifier", "Too few format specifiers", "Too many format specifiers", "Scan failed", "Newer CIN version", "Error converting to variant", "Runtime menu error", "Password tampered", "Variant attribute not found", "Incompatible variant data type", "Event data is not available", "Event Store is not present", "Occurrence is not found", "Event Queue is not created", "Event info is not available", "Refnum passed is NULL", "Error retrieving Class GUID", "Error retrieving CoClass GUID", "Error retrieving TypeLib GUID.", "Bad built application magic bytes.", "Specific driver is different from the specific driver associated with the Logical Name.", "There is no session opened to the class driver.", "Max Error", "MAX - Error with config objects", "MAX - Error loading configuration", "MAX - Group not supported"]
        # "Current State"
        # "Do not delete, rename, or modify this frame.\n(this is used to capture unhandled states and typos)"
        # "Handle mistyped state name (developer tool)"
        n144 = Format Into String(format string="Software Exception: Unhandled State \"%s\"." ("message"), error in=w252, w247) -> (resulting string=w255:string, error out=w254:errorcluster)  [unwired: 1 in]
        n145 = call <vilib>:"Error Cluster From Error Code.vi"("show call chain? (False)"=TRUE, "error in (no error)"=w254, "error message (\"\")"=w255, "error code (0)"=w256) -> ("error out"=w253:errorcluster)  [unwired: 5 in]
        n146 = call <vilib>:"Add State(s) to Queue__jki_lib_state_machine.vi"("State(s) in (\"\")"=w251) -> ("States Out"=w250:string)  [unwired: 14 in]
      }
      frame "Initialize Core Data" {
        # "Do not delete, rename, or modify this frame.\n(this is used to determine panel behavior on exit)"
        # "originally closed?"
        # "exe?"
        # "If panel starts closed or is an EXE, then close it when we exit"
        n147 = property class="VI"() -> ("Front Panel.Open"=w265:bool)  [unwired: 2 in, 2 out]
        n148 = property class="App"() -> ("App.Kind"=w264:T5)  [unwired: 2 in, 2 out]
        n149 = control-ref of="Current VI Reference"() -> (w258:refnum<vi>)
        n150 = Not(x=w265) -> (.not. x?=w262:bool)
        n151 = Equal?(x=w264, y=T5."Run Time System" ("Application:Kind")) -> (x = y?=w261:bool)
        n152 = Or(x=w262, y=w261) -> (x .or. y?=w259:bool)
        n153 = Bundle By Name(cluster=w260, "Core.Current VI Reference"=w258, "Core.Close Panel on Exit?"=w259) -> (w267:T10)
        n154 = call <vilib>:"Add State(s) to Queue__jki_lib_state_machine.vi"("State(s) in (\"\")"=w269) -> ("States Out"=w268:string)  [unwired: 14 in]
      }
      frame "Error Handler" {
        # "Unhandled Error -- Display it"
        # "Handle any errors here.\nYou can also output any states to clean-up after errors occur"
        # "Clear error"
        n155 = Wait (ms)(milliseconds to wait=u32 1500) -> ()  [unwired: 1 out]
        n156 = call <vilib>:"Add State(s) to Queue__jki_lib_state_machine.vi"("State(s) in Front (\"\")"="/* Post Error States", "State(s) in (\"\")"=w276) -> ("States Out"=w275:string)  [unwired: 13 in]
        "error out 5" <- w270
      }
      frame "Exit" {
        # "Do not put any code in this frame.\n(No errors that occur here will be handled.)"
        n157 = call <vilib>:"Add State(s) to Queue__jki_lib_state_machine.vi"("State(s) in (\"\")"=w281) -> ("States Out"=w280:string)  [unwired: 14 in]
      }
      frame "---------- Data ----------" {
        # "Do not put any code in this frame.\n(It is a separator no-op. You can make a copy of this frame to create a new Data frame)"
        n158 = call <vilib>:"Add State(s) to Queue__jki_lib_state_machine.vi"("State(s) in (\"\")"=w285) -> ("States Out"=w284:string)  [unwired: 14 in]
      }
      frame "Data: Initialize" {
        # "Initialize the shift-register data, here.\n(data names are defined by what you wire into the bundle function)"
        n159 = call "Data Cluster Plotter.vi"() -> ("output cluster"=w286:T10)
        n160 = call <vilib>:"Add State(s) to Queue__jki_lib_state_machine.vi"("State(s) in (\"\")"=w289) -> ("States Out"=w288:string)  [unwired: 14 in]
      }
      frame "Data: Cleanup" {
        # "Cleanup any data and references, here.\n(this is called automatically, by the Macro: Exit)"
        n161 = Unbundle By Name(w290) -> ("Core.Current VI Reference"=w293:refnum<vi>)
        n162 = Close Reference(reference=w293, error in (no error)=w292) -> (error out=w291:errorcluster)
        n163 = call <vilib>:"Add State(s) to Queue__jki_lib_state_machine.vi"("State(s) in (\"\")"=w295) -> ("States Out"=w294:string)  [unwired: 14 in]
      }
      frame "---------- UI ----------" {
        # "Do not put any code in this frame.\n(It is a separator no-op. You can make a copy of this frame to create a new UI frame)"
        n164 = call <vilib>:"Add State(s) to Queue__jki_lib_state_machine.vi"("State(s) in (\"\")"=w299) -> ("States Out"=w298:string)  [unwired: 14 in]
      }
      frame "UI: Initialize" {
        # "Initialize the User Interface, here.\n(this is called automatically, by the Macro: Init)"
        n165 = call <vilib>:"Add State(s) to Queue__jki_lib_state_machine.vi"("State(s) in (\"\")"=w303) -> ("States Out"=w302:string)  [unwired: 14 in]
      }
      frame "UI: Cursor Set" {
        # "Argument"
        # "Set and Unset Cursor Busy.\n(Usage: \"UI: Cursor Set >> Busy|Idle\")"
        n166 = case shown="\"Idle\", Default" w304 {
          tunnel: w306 -> [w311 w313]
          tunnel: [w310 w312] -> w305
          frame "Idle", Default {
            n167 = call <vilib>:"Unset Busy.vi"("error in (no error)"=w311) -> ("error out"=w310:errorcluster)  [unwired: 10 in]
          }
          frame "Busy" {
            n168 = call <vilib>:"Set Busy.vi"("error in (no error)"=w313) -> ("error out"=w312:errorcluster)  [unwired: 9 in, 1 out]
          }
        }
        n169 = call <vilib>:"Add State(s) to Queue__jki_lib_state_machine.vi"("State(s) in (\"\")"=w309) -> ("States Out"=w308:string)  [unwired: 14 in]
      }
      frame "UI: Front Panel State" {
        # "Argument"
        # "Set Front Panel Open or Closed\n(Usage: \"UI: Front Panel State >> Open|Close\")"
        n170 = Unbundle By Name(w316) -> ("Core.Current VI Reference"=w315:refnum<vi>)
        n171 = case shown="\"Open\", Default" w314 {
          tunnel: w318 -> [w324 w337]
          tunnel: [w326 w338] -> w317
          tunnel: w315 -> [w325 w335]
          frame "Open", Default {
            n172 = property class="VI"(reference=w325, error in=w324) -> (reference out=w322:refnum<vi>, error out=w323:errorcluster, "Front Panel.Open"=w321:bool)
            n173 = case shown="True" w321 {
              tunnel: [w329 w332] -> w326
              tunnel: w323 -> [w328 w332]
              tunnel: w322 -> [w327 _]
              frame False {
                n174 = invoke class="VI" method="FP.Open"(reference=w327, error in=w328, "Activate"=TRUE, "State"=T6."Standard") -> (error out=w329:errorcluster)  [unwired: 1 in, 4 out]
              }
              frame True {
              }
            }
          }
          frame "Close" {
            n175 = property class="VI"(reference=w335, error in=w337) -> (reference out=w334:refnum<vi>, error out=w336:errorcluster, "Front Panel.Open"=w333:bool)
            n176 = case shown="True" w333 {
              tunnel: [w339 w342] -> w338
              tunnel: w336 -> [w339 w341]
              tunnel: w334 -> [_ w340]
              frame False {
              }
              frame True {
                n177 = invoke class="VI" method="FP.Close"(reference=w340, error in=w341) -> (error out=w342:errorcluster)  [unwired: 1 in, 2 out]
              }
            }
          }
        }
        n178 = call <vilib>:"Add State(s) to Queue__jki_lib_state_machine.vi"("State(s) in (\"\")"=w320) -> ("States Out"=w319:string)  [unwired: 14 in]
      }
      frame "---------- Macro ----------" {
        # "Do not put any code in this frame.\n(It is a separator no-op. You can make a copy of this frame to create a new Macro frame)"
        n179 = call <vilib>:"Add State(s) to Queue__jki_lib_state_machine.vi"("State(s) in (\"\")"=w346) -> ("States Out"=w345:string)  [unwired: 14 in]
      }
      frame "Macro: Initialize" {
        w348 = "Data: Initialize\nInitialize Core Data\nUI: Initialize\nUI: Front Panel State >> Open\nMain: Macro"  # Data: Initialize Initialize Core Data UI: Initialize UI: Front Panel State >> Open Main: Macro
        # "Initialization Macro\n(This is called once, when the VI starts)"
        n180 = call <vilib>:"Add State(s) to Queue__jki_lib_state_machine.vi"("State(s) in Front (\"\")"=w348, "State(s) in (\"\")"=w351) -> ("States Out"=w350:string)  [unwired: 13 in]
      }
      frame "Macro: Exit" {
        # "Exit Macro\n(This is called once, when the VI exits)"
        n181 = Unbundle By Name(w359) -> ("Core.Close Panel on Exit?"=w358:bool)
        n182 = Select(t="UI: Front Panel State >> Close", s=w358, f="") -> (s? t:f=w355:string)
        n183 = call <vilib>:"Add State(s) to Queue__jki_lib_state_machine.vi"("State(s) in (\"\")"=w355, "State(s) at Back (\"\")"="Data: Cleanup\nExit") -> ("States Out"=w353:string)  [unwired: 13 in]
        n184 = call <vilib>:"Add State(s) to Queue__jki_lib_state_machine.vi"("State(s) in Front (\"\")"=w353, "State(s) in (\"\")"=w361) -> ("States Out"=w360:string)  [unwired: 13 in]
      }
      frame "---------- Main ----------" {
        # "Template Separator\n(You can make a copy of, or modify, this frame)"
        n185 = call <vilib>:"Add State(s) to Queue__jki_lib_state_machine.vi"("State(s) in (\"\")"=w365) -> ("States Out"=w364:string)  [unwired: 14 in]
      }
      frame "Main: Macro" {
        # "Sets the list of states to execute on vi startup in the first string and  the list of states to execute on each loop\nin the second string"
        n186 = local write "Tab Control"(0) -> ()
        n187 = call <vilib>:"Add State(s) to Queue__jki_lib_state_machine.vi"("State(s) in Front (\"\")"="Main: Read Expt Configs\nMain: Get Expt name\nGet plotter details\nMain: Read Expt Config\nGet List of Axis Names\nGet Default Y Axis\nMain: Set Panel Postion\nMain: Get Device Configs", "State(s) in (\"\")"=w371) -> ("States Out"=w370:string)  [unwired: 13 in]
      }
      frame "Main: Read Expt Configs" {
        # "Gets experimental configuration filenames. These files contain information specific to an experiment. Eg TREX expt\nfile would have all the devices that need to startup and their default variable values."
        n188 = call "preset SQL Queries.vi"("error in (no error)"=w373, "Preset Query"=Preset_Query_Enum."Get Expt names") -> ("error out"=w372:errorcluster, "1st column"=w374:string[])  [unwired: 7 in, 1 out]
        n189 = call "array to strings and values for ring.vi"("list of variables"=w374) -> ("Array"=w378:cluster{"String":string, i32}[])
        n190 = property on="Experiment" class="Ring (strict)"("StringsAndValues[]"=w378) -> ()  [unwired: 2 in, 2 out]
        n191 = Bundle By Name(cluster=w377, "Expt Config Files"=w374) -> (w376:T10)
        n192 = call <vilib>:"Add State(s) to Queue__jki_lib_state_machine.vi"("State(s) in (\"\")"=w380) -> ("States Out"=w379:string)  [unwired: 14 in]
      }
      frame "Main: Get Expt name" {
        # "cmd is ...plotter.exe>>plotterid#"
        # "Increments scan #, resets shot number and sends list of states to execute at the start of a scan. Only does this\nif variable for scan is numeric."
        n193 = disable-structure shown="RUN_TIME_ENGINE==True" {
          disable-tunnel: ["expt_Plotteridfor vi mode" w408] -> w381
          disable-tunnel: [_ w403] -> w385
          disable-tunnel: [_ w402] -> w383
          frame condition #0 (active) {
          }
          frame condition #1 {
            n194 = control-ref of="This Application"() -> (w409:refnum<vi>)
            n195 = property class="App"(reference=w409) -> ("App.Args"=w407:string[])  [unwired: 1 in, 2 out]
            "appargs" <- w407
            n196 = Index Array(array=w407, index #1=2 ("index"), index #2=3 ("index"), index #3=4 ("index")) -> (element #1=w408:string, element #2=w403:string, element #3=w402:string)
          }
        }
        "expt_plotter.id" <- w381
        n197 = Unbundle By Name(w398) -> ("Expt Config Files"=w396:string[])
        n198 = property on="Experiment" class="Ring (strict)"() -> ("Strings []"=w390:string[])  [unwired: 2 in, 2 out]
        n199 = call "preset SQL Queries.vi"("error in (no error)"=w387, "Device/Devicetype name\n/Plotter.id/#"=w381, "Preset Query"=Preset_Query_Enum."Get expt for plotter") -> ("error out"=w386:errorcluster, "data"=w393:string[][])  [unwired: 6 in, 1 out]
        n200 = Index Array(array=w393, index (row)=1) -> (element=w395:string[])  [unwired: 1 in]
        n201 = Decimal String To Number(string=w385) -> (number=w384:i32)  [unwired: 2 in, 1 out]
        n202 = Decimal String To Number(string=w383) -> (number=w382:i32)  [unwired: 2 in, 1 out]
        n203 = Index Array(array=w395) -> (element #1=w388:string, element #2=w391:string)  [unwired: 2 in]
        "expt" <- w388
        "plotter#" <- w391
        n204 = Search 1D Array(1D array=w390, element=w388) -> (index of element=w389:i32)  [unwired: 1 in]
        "Experiment" <- w389
        n205 = Index Array(array=w396, index=w389) -> ()  [unwired: 1 out]
        n206 = Bundle By Name(cluster=w398, "Experiment name"=w388, "plotter#"=w391, "Plotter setup cluster.screenx"=w384, "Plotter setup cluster.screeny"=w382) -> (w397:T10)
        n207 = call <vilib>:"Add State(s) to Queue__jki_lib_state_machine.vi"("State(s) in (\"\")"=w400) -> ("States Out"=w399:string)  [unwired: 14 in]
      }
      frame "Get plotter details" {
        # "Template Separator\n(You can make a copy of, or modify, this frame)"
        n208 = Unbundle By Name(w414) -> ("plotter#"=w424:string)
        n209 = call "preset SQL Queries.vi"("error in (no error)"=w411, "Device/Devicetype name\n/Plotter.id/#"=w424, "Preset Query"=Preset_Query_Enum."Get plotter details") -> ("error out"=w410:errorcluster, "data"=w423:string[][])  [unwired: 6 in, 1 out]
        "plotter details" <- w423
        n210 = Index Array(array=w423, index (row)=1) -> (element=w421:string[])  [unwired: 1 in]
        n211 = Index Array(array=w421) -> (element #2=w420:string, element #3=w418:string, element #4=w416:string, element #5=w415:string)  [unwired: 5 in, 1 out]
        n212 = Decimal String To Number(string=w420) -> (number=w419:i32)  [unwired: 2 in, 1 out]
        n213 = Decimal String To Number(string=w418) -> (number=w417:i32)  [unwired: 2 in, 1 out]
        n214 = Bundle By Name(cluster=T8 {"screenx"=25, "screeny"=75, "variable1"="", "variable2"=""} ("Plotter setup cluster"), "screenx"=w419, "screeny"=w417, "variable1"=w416, "variable2"=w415) -> (w412:T8)
        n215 = Bundle By Name(cluster=w414, "Plotter setup cluster"=w412) -> (w413:T10)
        n216 = call <vilib>:"Add State(s) to Queue__jki_lib_state_machine.vi"("State(s) in (\"\")"=w428) -> ("States Out"=w427:string)  [unwired: 14 in]
      }
      frame "Main: Read Expt Config" {
        # "todo. get rid of the copy of parameters"
        # "Reads the configuration for a particular experiment. eg TREX default would save spectrum mode image and\nget back centroid etc."
        n217 = Unbundle By Name(w455) -> ("Experiment name"=w437:string)
        n218 = call "preset SQL Queries.vi"("error in (no error)"=w436, "Expt name / MCIP/ Variable Name"=w437, "Preset Query"=Preset_Query_Enum."Get experiment basic properties") -> ("error out"=w435:errorcluster, "1st column"=w433:string[], "data"=w432:string[][])  [unwired: 6 in]
        n219 = Index Array(array=w433) -> (element=w439:string)  [unwired: 1 in]
        n220 = Index Array(array=w432, index (row)=1, index (col)=2 ("disabled index (col)")) -> (element=w429:string)
        n221 = call "preset SQL Queries.vi"("error in (no error)"=w435, "Expt name / MCIP/ Variable Name"=w437, "Preset Query"=Preset_Query_Enum."Get expt devices with data to get") -> ("error out"=w453:errorcluster, "data"=w450:string[][])  [unwired: 6 in, 1 out]
        n222 = Decimal String To Number(string=w429) -> (number=w434:i32)  [unwired: 2 in, 1 out]
        n223 = Delete From Array(array=w450, index (row)=0) -> (array with subset deleted=w452:string[][])  [unwired: 2 in, 1 out]
        n224 = Index Array(array=w452, index (col)=0 ("disabled index (col)")) -> (element=w445:string[])  [unwired: 1 in]
        "devices to get data from" <- w445
        n225 = call "preset SQL Queries.vi"("error in (no error)"=w453, "Expt name / MCIP/ Variable Name"=w437, "Preset Query"=Preset_Query_Enum."Get expt devices and variables (with data to get)") -> ("error out"=w446:errorcluster, "data"=w444:string[][])  [unwired: 6 in, 1 out]
        "parameters to get" <- w444
        n226 = Bundle By Name(cluster=w455, "expt config file array"=w444, "ScanData to receive"=w444, "Device Names for scan data"=w445) -> (w454:T10)
        n227 = call "Plotter FGV Cluster.vi"("Function"=enum16{"Read", "Write", "Clear"}."Read") -> ("Cluster out"=w440:T4)  [unwired: 9 in, 1 out]
        n228 = Bundle By Name(cluster=w440, "Multicast Address"=w439, "Mcast Port"=w434) -> (w438:T4)
        n229 = call <vilib>:"Add State(s) to Queue__jki_lib_state_machine.vi"("State(s) in (\"\")"=w457) -> ("States Out"=w456:string)  [unwired: 14 in]
        n230 = call "Plotter FGV Cluster.vi"("Function"=enum16{"Read", "Write", "Clear"}."Write", "Cluster in"=w438) -> ()  [unwired: 8 in, 2 out]
      }
      frame "Get List of Axis Names" {
        # "Increments scan #, resets shot number and sends list of states to execute at the start of a scan. Only does this\nif variable for scan is numeric."
        n231 = Unbundle By Name(w463) -> ("ScanData to receive"=w461:string[][])
        n232 = Delete From Array(array=w461, index (row)=0) -> (array with subset deleted=w459:string[][])  [unwired: 2 in, 1 out]
        n233 = Index Array(array=w459, index (col) #1=0 ("disabled index (col)"), index (col) #2=1 ("index (col)")) -> (element #1=w465:string[], element #2=w464:string[])  [unwired: 2 in]
        n234 = for {
          tunnel: w465 -> [w473] mode=indexing
          tunnel: w464 -> [w472] mode=indexing
          tunnel: [w471] -> w458 mode=indexing
          n235 = Concatenate Strings(w473, " " ("string"), w472) -> (w471:string)
        }
        "Axis Name List" <- w458
        n236 = Bundle By Name(cluster=w463, "Data titles from config array"=w458) -> (w462:T10)
        n237 = property on="Y Axis 2" class="Ring (strict)"("Strings []"=w458) -> ()  [unwired: 2 in, 2 out]
        n238 = property on="Y Axis" class="Ring (strict)"("Strings []"=w458) -> ()  [unwired: 2 in, 2 out]
        n239 = property on="X Axis" class="Ring (strict)"("Strings []"=w458) -> ()  [unwired: 2 in, 2 out]
        n240 = call <vilib>:"Add State(s) to Queue__jki_lib_state_machine.vi"("State(s) in (\"\")"=w470) -> ("States Out"=w469:string)  [unwired: 14 in]
      }
      frame "Get Default Y Axis" {
        # "Increments scan #, resets shot number and sends list of states to execute at the start of a scan. Only does this\nif variable for scan is numeric."
        n241 = Unbundle By Name(w483) -> ("Plotter setup cluster.variable1"=w478:string, "Plotter setup cluster.variable2"=w477:string)
        "Y Axis Default name" <- w478
        n242 = stacked-sequence {
          tunnel: w478 -> [w490 w494]
          tunnel: w477 -> [w489 w493]
          tunnel: 0 ("Active Y Scale") -> [w488 w492]
          tunnel: 1 ("Active Y Scale") -> [w487 w491]
          frame #0 {
            n243 = property on="xy graph" class="XYGraph (strict)"("ActYScl"=w488, "YScale.NameLbl.Text"=w490, "ActYScl"=w487, "YScale.NameLbl.Text"=w489) -> ()  [unwired: 2 in, 2 out]
          }
          frame #1 {
            n244 = property on="xy graph bin" class="XYGraph (strict)"("ActYScl"=w492, "YScale.NameLbl.Text"=w494, "ActYScl"=w491, "YScale.NameLbl.Text"=w493) -> ()  [unwired: 2 in, 2 out]
          }
        }
        n245 = property on="Y Axis" class="Ring (strict)"() -> ("Strings []"=w482:string[])  [unwired: 2 in, 2 out]
        n246 = property on="Y Axis 2" class="Ring (strict)"() -> ("Strings []"=w480:string[])  [unwired: 2 in, 2 out]
        n247 = Search 1D Array(1D array=w480, element=w477) -> (index of element=w479:i32)  [unwired: 1 in]
        n248 = Search 1D Array(1D array=w482, element=w478) -> (index of element=w481:i32)  [unwired: 1 in]
        n249 = local write "Y Axis"(w481) -> ()
        n250 = local write "Y Axis 2"(w479) -> ()
        n251 = call <vilib>:"Add State(s) to Queue__jki_lib_state_machine.vi"("State(s) in (\"\")"=w486) -> ("States Out"=w485:string)  [unwired: 14 in]
      }
      frame "open tcp connections" {
        # "Your code here.\n(You can make a copy of, or modify, this frame)"
        n252 = disable-structure shown="Enabled" {
          disable-tunnel: w499 -> [w529 w550]
          disable-tunnel: w498 -> [w509 _]
          disable-tunnel: [w508 _] -> w497
          disable-tunnel: [w504 w547] -> w496
          disable-tunnel: [w508 _] -> w495
          frame Enabled {
            w503 = "Shot #" ("Active Variable")
            w511 = 1000 ("timeout ms (60000)")
            n253 = local read "x axis name"() -> (w506:string)
            n254 = Unbundle By Name(w529) -> ("Plotter setup cluster.variable1"=w528:string, "Plotter setup cluster.variable2"=w523:string)
            n255 = Equal?(x=w506, y=w503) -> (x = y?=w507:bool)
            "shotoverride" <- w507
            n256 = Search/Split String(string=w528, search string/char (-)=" ") -> (substring before match=w526:string, match + rest of string=w525:string)  [unwired: 1 in, 1 out]
            n257 = call "subscribe command.vi"("variable"=w523) -> ("IP"=w521:string, "port"=w519:string, "subscribe command"=w513:string)
            n258 = String Subset(string=w525, offset (0)=1) -> (substring=w515:string)  [unwired: 1 in]
            n259 = call "get device ip and port.vi"("variable1"=w526) -> ("port"=w520:string, "IP"=w522:string)  [unwired: 1 out]
            n260 = Build Array(w522, w521) -> (w518:string[])
            "ipjjj" <- w518
            n261 = Build Array(w520, w519) -> (w517:string[])
            "portrsvvv" <- w517
            n262 = Concatenate Strings("Wait>>" ("search string/char (-)"), w515) -> (w514:string)
            n263 = call "TCP multiple open.vi"("timeout ms (60000)"=w511, "Ports"=w517, "error in 1 (no error)"=w509, "IP Addresses"=w518) -> ("error out"=w510:errorcluster, "Array"=w505:refnum<k5>[])  [unwired: 1 out]
            n264 = case shown="False" w507 {
              tunnel: w506 -> [w530 _]
              tunnel: [w531 w546] -> w504
              tunnel: w505 -> [w533 w546]
              tunnel: w503 -> [_ w545]
              frame False {
                w534 = 1000 ("timeout ms (60000)")
                n265 = call "subscribe command.vi"("variable"=w530) -> ("IP"=w541:string, "port"=w542:string, "subscribe command"=w535:string)
                "subscribe command" <- w535
                n266 = Decimal String To Number(string=w542) -> (number=w544:i32)  [unwired: 2 in, 1 out]
                n267 = property on="xy graph" class="XYGraph (strict)"("XScale.NameLbl.Text"=w530) -> ()  [unwired: 2 in, 2 out]
                n268 = To Unsigned Word Integer(number=w544) -> (unsigned 16bit integer=w543:u16)
                n269 = TCP Open Connection(address=w541, remote port or service name=w543, timeout ms (60000)=w534) -> (connection ID=w536:refnum<k5>)  [unwired: 2 in, 1 out]
                n270 = String Length(string=w535) -> (length=w539:i32)
                n271 = Type Cast(type=w535, x=w539) -> (*(type *) &x=w540:string)
                n272 = TCP Write(connection ID=w536, data in=w540) -> (connection ID out=w537:refnum<k5>, error out=w538:errorcluster)  [unwired: 2 in, 1 out]
                n273 = TCP Write(connection ID=w537, data in=w535, error in (no error)=w538, 9:w534) -> (connection ID out=w532:refnum<k5>)  [unwired: 2 out]
                n274 = Build Array (concatenate)(w533, w532) -> (w531:refnum<k5>[])
              }
              frame True {
                n275 = property on="xy graph" class="XYGraph (strict)"("XScale.NameLbl.Text"=w545) -> ()  [unwired: 2 in, 2 out]
                n276 = local write "x axis name"(w545) -> ()
                n277 = property on="xy graph bin" class="XYGraph (strict)"("XScale.NameLbl.Text"=w545) -> ()  [unwired: 2 in, 2 out]
              }
            }
            n278 = Build Array(w514, w513) -> (w512:string[])
            "appended array" <- w512
            n279 = call "tcp multiple write.vi"("Connection ID array"=w505, "error in 1 (no error)"=w510, "messages to send"=w512, "timeout ms (25000)"=w511) -> ("error out"=w508:errorcluster)
          }
          frame Disabled {
            n280 = Unbundle By Name(w550) -> ("All Devices Core Info"=w549:string[][], "Device Names for scan data"=w548:string[], "ScanData to receive"=w558:string[][])
            "ScanData to receive" <- w558
            n281 = call "get info from core device data.vi"("devices to get data from"=w548, "All Devices Core Info"=w549) -> ("Ports"=w557:string[], "IP Addresses"=w551:string[])  [unwired: 2 in]
            "udp ports to listen to" <- w557
            "IPs" <- w551
            n282 = call "scan data to receive to subscribe commands.vi"("ScanData to receive"=w558) -> ("Subscribe commands"=w556:string[])  [unwired: 9 in, 1 out]
            n283 = call "TCP multiple open.vi"("timeout ms (60000)"="TCP Open timeout ms", "Ports"=w557, "IP Addresses"=w551) -> ("error out"=w553:errorcluster, "Array"=w547:refnum<k5>[])  [unwired: 1 in]
            n284 = call "tcp multiple write.vi"("Connection ID array"=w547, "error in 1 (no error)"=w553, "messages to send"=w556, "timeout ms (25000)"=300) -> ("error out"=→"TCP scan error out":errorcluster)
          }
        }
        n285 = case shown="Error" w495 {
          tunnel: w496 -> [w502 _]
          frame No Error {
            "TCP Ports" <- w502
          }
          frame Error {
          }
        }
        n286 = call <vilib>:"Add State(s) to Queue__jki_lib_state_machine.vi"("State(s) in (\"\")"=w501) -> ("States Out"=w500:string)  [unwired: 14 in]
      }
      frame "Main: Set Panel Postion" {
        # "Reads the configuration for a particular experiment. eg TREX default would save spectrum mode image and\nget back centroid etc."
        n287 = Unbundle By Name(w568) -> ("Plotter setup cluster.screenx"=w564:i16, "Plotter setup cluster.screeny"=w563:i16)
        n288 = property on="Tab Control" class="TabCtl (strict)"() -> ("PaneWidth"=w572:u32, "PaneHeight"=w571:u32)  [unwired: 2 in, 2 out]
        n289 = Add(x=w571, y=u32 25) -> (x+y=w561:u32)
        n290 = Add(x=u32 15, y=w572) -> (x+y=w562:u32)
        n291 = call <vilib>:"Add State(s) to Queue__jki_lib_state_machine.vi"("State(s) in (\"\")"=w574) -> ("States Out"=w573:string)  [unwired: 14 in]
        n292 = Bundle By Name(cluster="Cluster", "Left"=w564, "Top"=w563, "Width"=w562, "Height"=w561) -> (w566:T1)
        n293 = control-ref of="This VI"() -> (w565:refnum<vi>)
        n294 = call "set panel position MC only.vi"("error out 2"=w560, "Cluster"=w566, "This VI"=w565) -> ("error out"=w559:errorcluster)
      }
      frame "Main: Get Device Configs" {
        # "Reads the configuration for a particular experiment. eg TREX default would save spectrum mode image and\nget back centroid etc."
        n295 = call "preset SQL Queries.vi"("error in (no error)"=w576, "Preset Query"=Preset_Query_Enum."Get all devices basic properties") -> ("error out"=w575:errorcluster, "data"=w577:string[][])  [unwired: 7 in, 1 out]
        "All Devices Core Info" <- w577
        n296 = Bundle By Name(cluster=w579, "All Devices Core Info"=w577) -> (w580:T10)
        n297 = call <vilib>:"Add State(s) to Queue__jki_lib_state_machine.vi"("State(s) in (\"\")"=w582) -> ("States Out"=w581:string)  [unwired: 14 in]
      }
      frame "Plot" {
        # "Your code here.\n(You can make a copy of, or modify, this frame)"
        n298 = Unbundle By Name(w605) -> ("TDMS file path"=w603:path)
        "TDMS file path" <- w603
        n299 = call "Plotter FGV Cluster.vi"("error in"=w586, "Function"=enum16{"Read", "Write", "Clear"}."Read") -> ("error out"=w594:errorcluster, "Cluster out"=w596:T4)  [unwired: 8 in]
        n300 = Bundle By Name(cluster=w596, "Plotter Busy"=TRUE) -> (w593:T4)
        n301 = Select(t="file path", s="FilePath", f=w603) -> (s? t:f=w602:path)
        "Path used" <- w602
        n302 = call "Plotter FGV Cluster.vi"("error in"=w594, "Function"=enum16{"Read", "Write", "Clear"}."Write", "Cluster in"=w593) -> ("error out"=w598:errorcluster, "Cluster out"=w589:T4)  [unwired: 7 in]
        n303 = Bundle By Name(cluster=w589, "Plotter Busy"=FALSE) -> (w588:T4)
        n304 = call <vilib>:"Check if File or Folder Exists.vi"("error in (no error)"=w598, "path"=w602) -> ("error out"=w599:errorcluster, "file or folder exists?"=w601:bool, "dup path"=w600:path)  [unwired: 7 in]
        n305 = case shown="True" w601 {
          tunnel: w600 -> [_ w617]
          tunnel: w605 -> [_ w620]
          tunnel: w599 -> [w608 w616]
          tunnel: [w608 w616] -> w590
          tunnel: w584 -> [_ w619]
          tunnel: "FilePath" -> [_ w618]
          frame False {
          }
          frame True {
            n306 = local read "shot# 2"() -> (w610:i32)
            n307 = local read "y2"() -> (w614:dbl[])
            n308 = local read "y1"() -> (w612:dbl[])
            n309 = Array Subset(array=w612, index=1, length=w610) -> (w609:dbl[])
            n310 = Array Subset(array=w614, index=1, length=w610) -> (w613:dbl[])
            n311 = stacked-sequence {
              tunnel: w617 -> [w626 _ _ w646 w683]
              tunnel: w620 -> [_ w637 _ _ w682]
              tunnel: w619 -> [_ _ _ _ w684]
              tunnel: w618 -> [_ _ _ w644 _]
              tunnel: w613 -> [w621 _ _ w643 _]
              tunnel: w609 -> [_ _ _ w642 _]
              frame #0 {
                n312 = Array Size(array=w621) -> (size(s)=w625:i32)
                n313 = In Range and Coerce(upper limit=4 ("y"), x=w625, lower limit=2) -> (In Range?=w623:bool)  [unwired: 1 out]
                n314 = case shown="True" w623 {
                  tunnel: w626 -> [_ w627]
                  frame False {
                  }
                  frame True {
                    n315 = call "Read TDMS - LOASIS scan data.vi"("file path"=w627) -> ("device data Spreadsheet format"=w630:string[][])  [unwired: 9 in, 1 out]
                    n316 = Index Array(array=w630, index (row)=0) -> (element=w628:string[])  [unwired: 1 in]
                    n317 = property on="Y Axis 2" class="Ring (strict)"("Strings []"=w628) -> ()  [unwired: 2 in, 2 out]
                    n318 = property on="X Axis" class="Ring (strict)"("Strings []"=w628) -> ()  [unwired: 2 in, 2 out]
                    n319 = property on="Y Axis" class="Ring (strict)"("Strings []"=w628) -> ()  [unwired: 2 in, 2 out]
                  }
                }
              }
              frame #1 {
                n320 = Unbundle By Name(w637) -> ("Plotter setup cluster.variable1"=w635:string, "Plotter setup cluster.variable2"=w632:string)
                n321 = property on="Y Axis 2" class="Ring (strict)"() -> ("Strings []"=w633:string[])  [unwired: 2 in, 2 out]
                n322 = property on="Y Axis" class="Ring (strict)"() -> ("Strings []"=w636:string[])  [unwired: 2 in, 2 out]
                n323 = Search 1D Array(1D array=w633, element=w632) -> (index of element=w631:i32)  [unwired: 1 in]
                n324 = Search 1D Array(1D array=w636, element=w635) -> (index of element=w634:i32)  [unwired: 1 in]
                n325 = local write "Y Axis 2"(w631) -> ()
                n326 = local write "Y Axis"(w634) -> ()
              }
              frame #2 {
                n327 = local read "FilePath"() -> (w638:bool)
                n328 = case shown="False" w638 {
                  frame False {
                    n329 = local read "x axis name"() -> (w640:string)
                    n330 = property on="X Axis" class="Ring (strict)"() -> ("Strings []"=w641:string[])  [unwired: 2 in, 2 out]
                    n331 = Search 1D Array(1D array=w641, element=w640) -> (index of element=w639:i32)  [unwired: 1 in]
                    n332 = local write "X Axis"(w639) -> ()
                  }
                  frame True {
                  }
                }
              }
              frame #3 {
                n333 = case shown="False" w644 {
                  tunnel: w646 -> [_ w670]
                  tunnel: [w662 w678] -> w645
                  tunnel: w643 -> [w651 _]
                  tunnel: w642 -> [w648 _]
                  frame False {
                    w647 = 1000 ("max array size")
                    n334 = local read "shotoverride"() -> (w660:bool)
                    n335 = local read "shot# 2"() -> (w657:i32)
                    n336 = local read "shot#"() -> (w658:i32)
                    n337 = Greater?(x=w658, y=w657) -> (0:w659:bool)
                    n338 = Select(t=w658, s=w659, f=w657) -> (s? t:f=w656:i32)
                    n339 = case shown="True" w660 {
                      tunnel: [w663 w668] -> w661
                      tunnel: w656 -> [_ w667]
                      frame False {
                        n340 = local read "x"() -> (w666:dbl[])
                        n341 = Delete From Array(array=w666, length=1, index=0) -> (array with subset deleted=w663:dbl[])  [unwired: 1 out]
                      }
                      frame True {
                        n342 = call-poly <vilib>:"Ramp Pattern.vi"("start"=1.0, "end"=w667, "samples"=w667) -> ("Ramp Pattern"=w668:dbl[])  [unwired: 7 in, 1 out]
                      }
                    }
                    n343 = call <vilib>:"Std Deviation and Variance.vi"("X"=w651) -> ("mean"=→"RHS mean":dbl, "standard deviation"=→"RHS sigma":dbl)  [unwired: 1 in, 1 out]
                    n344 = call "decimate array max points.vi"("max array size"=w647, "Array in"=w651) -> ("Decimated Array out"=w650:dbl[])  [unwired: 9 in]
                    n345 = call "decimate array max points.vi"("max array size"=w647, "Array in"=w648) -> ("Decimated Array out"=w649:dbl[])  [unwired: 9 in]
                    n346 = call <vilib>:"Std Deviation and Variance.vi"("X"=w648) -> ("mean"=→"LHS mean":dbl, "standard deviation"=→"LHS sigma":dbl)  [unwired: 1 in, 1 out]
                    n347 = call "xy graph from 1d arrays.vi"("y2"=w650, "y1"=w649, "shot#"=w656, "x"=w661) -> ("xy graph"=w662:cluster{"Ramp Pattern":dbl[], dbl[]}[])
                  }
                  frame True {
                    n348 = control-ref of="XY Graph"() -> (w677:refnum<vi>)
                    n349 = control-ref of="Y Axis 2"() -> (w676:refnum<vi>)
                    n350 = call "Read TDMS - LOASIS scan data.vi"("file path"=w670) -> ("device data Spreadsheet format"=w671:string[][])  [unwired: 9 in, 1 out]
                    n351 = control-ref of="Y Axis"() -> (w675:refnum<vi>)
                    n352 = control-ref of="X Axis"() -> (w674:refnum<vi>)
                    n353 = Bundle By Name(cluster=T9 {"Ring Refnum x"=refnum, "Ring Refnum y"=refnum, "Ring Refnum y 2"=refnum, "XY Graph Refnum"=refnum} ("Cluster"), "Ring Refnum x"=w674, "Ring Refnum y"=w675, "Ring Refnum y 2"=w676, "XY Graph Refnum"=w677) -> (w672:T9)
                    n354 = call "Select axes.vi"("Cluster"=w672, "output array"=w671) -> ("XY Graph"=w678:cluster{dbl[], dbl[]}[])  [unwired: 4 in, 2 out]
                  }
                }
                "xy graph" <- w645
              }
              frame #4 {
                # "todo. use multiple bin"
                n355 = Unbundle By Name(w682) -> ("Plotter setup cluster.variable1"=w680:string, "Plotter setup cluster.variable2"=w681:string)
                n356 = local read "x axis name"() -> (w679:string)
                n357 = case shown="\"bin\"" w684 {
                  tunnel: w683 -> [_ w686]
                  tunnel: w681 -> [_ w689]
                  tunnel: w680 -> [_ w688]
                  tunnel: w679 -> [_ w687]
                  frame "nobin", Default {
                  }
                  frame "bin" {
                    n358 = call "Read TDMS - LOASIS scan data.vi"("file path"=w686) -> ("device data Spreadsheet format"=w685:string[][])  [unwired: 9 in, 1 out]
                    "device data Spreadsheet format" <- w685
                    n359 = call "binning for loasis TDMS plotter.vi"("y2 col name"=w689, "y1 col name"=w688, "x col name"=w687, "device data Spreadsheet format"=w685) -> ("xy graph bin"=→"xy graph bin":cluster{dbl[], dbl[]}[])  [unwired: 7 in]
                  }
                }
              }
            }
          }
        }
        n360 = call "Plotter FGV Cluster.vi"("error in"=w590, "Function"=enum16{"Read", "Write", "Clear"}."Write", "Cluster in"=w588) -> ("error out"=w585:errorcluster)  [unwired: 7 in, 1 out]
        n361 = call <vilib>:"Add State(s) to Queue__jki_lib_state_machine.vi"("State(s) in (\"\")"=w607) -> ("States Out"=w606:string)  [unwired: 14 in]
      }
      frame "19" {
        # "Your code here.\n(You can make a copy of, or modify, this frame)"
        n362 = call <vilib>:"Add State(s) to Queue__jki_lib_state_machine.vi"("State(s) in (\"\")"=w694) -> ("States Out"=w693:string)  [unwired: 14 in]
      }
    }
    "error out 2" <- w138
  }
  n363 = stacked-sequence "TCP subsrcriptions for scan data" {
    tunnel: w1 -> [_ w699]
    frame #0 {
      n364 = local write "TCP Ports"(refnum<k5>[] [] ("TCP Ports")) -> ()
    }
    frame #1 {
      n365 = control-ref of="shot#"() -> (w702:refnum<vi>)
      n366 = control-ref of="TCP Ports"() -> (w704:refnum<vi>)
      n367 = control-ref of="y1"() -> (w703:refnum<vi>)
      n368 = control-ref of="data out 1"() -> (w697:refnum<vi>)
      n369 = Bundle("TCP Ports"=w704, "y1"=w703, "shot#"=w702, "data out 1"=w697) -> (w701:T11)  [unwired: 1 in]
      n370 = call "Plotter TCP Reader1.vi"("error in"=w699, "timeout ms"="timeout ms", "TCP index"=0, "references"=w701) -> ("error out"=→"error out":errorcluster)  [unwired: 7 in]
    }
  }
  n371 = stacked-sequence "TCP subsrcriptions for scan data" {
    tunnel: w1 -> [_ w710]
    frame #0 {
      n372 = local write "TCP Ports"(refnum<k5>[] [] ("TCP Ports")) -> ()
    }
    frame #1 {
      n373 = control-ref of="TCP Ports"() -> (w714:refnum<vi>)
      n374 = control-ref of="shot# 2"() -> (w712:refnum<vi>)
      n375 = control-ref of="y2"() -> (w713:refnum<vi>)
      n376 = control-ref of="data out 2"() -> (w711:refnum<vi>)
      n377 = Bundle("TCP Ports"=w714, "y2"=w713, "shot# 2"=w712, "data out 2"=w711) -> (w709:T12)  [unwired: 1 in]
      n378 = call "Plotter TCP Reader2.vi"("error in"=w710, "timeout ms"=1000, "TCP index"=1, "references"=w709) -> ("error out"=→"error out 3":errorcluster)  [unwired: 7 in]
    }
  }
  n379 = stacked-sequence "TCP subsrcriptions for scan data" {
    tunnel: w1 -> [_ w718]
    frame #0 {
      n380 = local write "TCP Ports"(refnum<k5>[] [] ("TCP Ports")) -> ()
    }
    frame #1 {
      n381 = control-ref of="TCP Ports"() -> (w722:refnum<vi>)
      n382 = control-ref of="x"() -> (w723:refnum<vi>)
      n383 = control-ref of="data out 3"() -> (w724:refnum<vi>)
      n384 = control-ref of="shot# 3"() -> (w716:refnum<vi>)
      n385 = Bundle("TCP Ports"=w722, "x"=w723, "shot# 3"=w716, "data out 3"=w724) -> (w721:T13)  [unwired: 1 in]
      n386 = call "Plotter TCP Reader3.vi"("error in"=w718, "timeout ms"=1000, "TCP index"=2, "references"=w721) -> ("error out"=→"error out 4":errorcluster)  [unwired: 7 in]
    }
  }
